vi "01 Dryer Start Stop SM.vi"() -> ()   [LabVIEW 2012]
uses:
  Dryer Com Port Info.ctl
  Dryer Status Ctrl.ctl
  StartStop Data.ctl
  GEA2 Driver/GEA2 Dryer Interface Ctrl.ctl
  <vilib>/DAQmx/read.llb/DAQmx Read (Analog 2D DBL NChan NSamp).vi
  <vilib>/DAQmx/write.llb/DAQmx Write (Digital U32 1Chan 1Samp).vi
  <vilib>/DAQmx/create/channels.llb/DAQmx Create Channel (AI-Voltage-Basic).vi
  <vilib>/DAQmx/configure/timing.llb/DAQmx Timing (Sample Clock).vi
  <vilib>/DAQmx/miscellaneous.llb/DAQmx Fill In Error Info.vi
  Globals SS.vi
  <vilib>/DAQmx/create/channels.llb/DAQmx Create Channel (DO-Digital Output).vi
  <vilib>/Utility/file.llb/Read From Spreadsheet File (DBL).vi
  <vilib>/Utility/file.llb/Write To Spreadsheet File (string).vi
  <vilib>/Utility/file.llb/Write To Spreadsheet File (DBL).vi
panel:
  in  "Tab Control":T1(tab)=enum."Raw Data"
  in  "D Data 2":dbl[](array[numeric])=[0.06788055309111314, 0.06788055309111314, 0.06788055309111314, 0.06788055309111314, 0.06788055309111314, 0.06788055309111314, 0.06788055309111314, 0.06788055309111314, 0.06788055309111314, 0.06788055309111314, 0.06788055309111314, 0.06788055309111314, 0.06788055309111314, 0.06788055309111314, 0.06788055309111314]
  in  "A Data 2":dbl[](array[numeric])
  in  "A Data":dbl[](array[numeric])
  in  "B Data":dbl[](array[numeric])
  in  "B Data 2":dbl[](array[numeric])
  in  "C Data 2":dbl[](array[numeric])
  in  "C Data":dbl[](array[numeric])
  in  "D Data":dbl[](array[numeric])=[5.851428694297497, 3.661927497414327, 3.661927497414327, 3.661927497414327, 3.661927497414327, 3.661927497414327, 3.661927497414327, 3.661927497414327, 3.661927497414327, 0.6577281807606751, 0.09762322341846881, 0.09762322341846881, 0.09762322341846881, 0.09762322341846881, 0.09762322341846881]
  in  "A save":dbl[](array[numeric])
  in  "C save":dbl[](array[numeric])
  in  "B save":dbl[](array[numeric])
  in  "D save":dbl[](array[numeric])=[5.851428694297497, 3.661927497414327, 3.661927497414327, 3.661927497414327, 3.661927497414327, 3.661927497414327, 3.661927497414327, 3.661927497414327, 3.661927497414327, 0.6577281807606751, 0.09762322341846881, 0.09762322341846881, 0.09762322341846881, 0.09762322341846881, 0.09762322341846881]
  out "Waveform Chart":dbl(graph)=0.09762322341846881
  in  "Channel":i32=6
  out "Currents":dbl[](array[numeric])=[0.0012165306634386985, -0.006587335189708488, 0.00045533310115012174, 0.009590983127054642, 0.09094609304713201, 0.048033305281516, 0.09762322341846881, 0.06788055309111314] format="%0.2f"
  in  "AI Task":refnum<k21>
  in  "Maximum Value":dbl=10.0 format="%0.2f"
  in  "Minimum Value":dbl=-10.0 format="%0.2f"
  in  "Rate":dbl=2.0 caption="Sample Rate (Hz)" format="%0.2f"
  in  "Samples per Channel":i32=1
  out "data":dbl[][](array[numeric])=[[0.0002433061326877397], [-0.0013174670379416976], [9.106662023002435e-05], [0.0019181966254109284], [0.018189218609426402], [0.0096066610563032], [0.019524644683693762], [0.013576110618222628]] format="%0.2f"
  in  "AI Channel":string="Dev2/ai0:7"
  out "Current State":string="Exit"
  out "Saving":errorcluster
  out "Stop":bool=TRUE
  out "Read Serial Count":dbl=792.0
  out "Log Coms Array":string[](array[string])=["COM2,3/1/2012,10:47:12 AM,No Com", "COM3,3/1/2012,10:47:12 AM,No Com", "COM4,3/1/2012,10:47:12 AM,No Com", "COM5,3/1/2012,10:47:12 AM,"]
  out "Status Array Out":T2[](array[typedef])=[{"Color"=0, "Last Read Status"=enum."Err", "Command:Data"="No Com", "Com Port"=2, "Time(S)"=158.546875, "Err Count"=233}, {"Color"=0, "Last Read Status"=enum."Err", "Command:Data"="No Com", "Com Port"=3, "Time(S)"=158.546875, "Err Count"=233}, {"Color"=0, "Last Read Status"=enum."Err", "Command:Data"="No Com", "Com Port"=4, "Time(S)"=158.5625, "Err Count"=233}, {"Color"=6618880, "Last Read Status"=enum."Cycle Running", "Command:Data"="", "Com Port"=5, "Time(S)"=158.5625, "Err Count"=1}]
  out "Rising Edge Out":bool[](array[boolean])
  in  "Power":bool[](array[boolean])=[FALSE, FALSE, FALSE, FALSE]
  in  "Power Port":tag="Dev2/port0" caption="Port"
  out "Restart Err Count":dbl=1.0
  in  "Cycle Save Multiple":i16=25
  out "Com Er Mess":string="Send Restart"
  out "Label Com Array":string[][](array[string])=[["Dryer A", "2"], ["Dryer B", "3"], ["Dryer C", "4"], ["Dryer D", "5"]]
  out "Current Filename":path=path "C:/Data/20120301_10_CONWAY-E5500.appl.ge.com_Dryer A_SS_Data.csv"
  in  "Timeout":i32=500
  in  "Config File":path=path "C:/data/SS_Config.ini"
  in  "Save File Path":path=path "C:/Data/Start Stop"
  out "robo?":bool
  out "Computer Name":string="CONWAY-E5500.appl.ge.com"
  in  "Cycle Count Path":path=path "c:/Data/CycleCount.csv"
  in  "Backup Hour":string="4"
  in  "Up Lim":dbl[](array[numeric])=[50.0, 50.0, 50.0, 50.0, 50.0, 4.4, 4.4, 50.0, 50.0, 50.0, 50.0, 1.0, 1.0, 1.0, 50.0, 50.0, 50.0, 50.0, 50.0, 50.0, 27.0, 27.0, 27.0, 27.0, 27.0, 27.0, 27.0, 27.0, 1.0, 1.0, 1.0, 1.0]
  in  "Low Lim 2":dbl[](array[numeric])=[-1.0, -1.0, -1.0, -1.0, -1.0, 3.5, 3.5, -1.0, -1.0, -1.0, -1.0, -1.0, -1.0, -1.0, -1.0, -1.0, -1.0, -1.0, -1.0, -1.0, -1.0, -1.0, -1.0, 22.0, -1.0, -1.0, -1.0, -1.0, -1.0, -1.0, -1.0, -1.0]
  in  "Low Lim":dbl[](array[numeric])=[-1.0, -1.0, -1.0, -1.0, -1.0, 3.5, 3.5, -1.0, -1.0, -1.0, -1.0, -1.0, -1.0, -1.0, -1.0, -1.0, -1.0, -1.0, -1.0, -1.0, -1.0, -1.0, 22.0, -1.0, -1.0, -1.0, -1.0, -1.0, -1.0, -1.0, -1.0, -1.0]
  in  "Off On Threshold":dbl=1.0
  in  "Filename Currents":path=path "c:/Data/Currents.csv"
  out "Max Len":i32
  out "A Array":string[][](array[string])
  out "B Array":string[][](array[string])
  out "D Array":string[][](array[string])=[["Dryer D,COM5,3/1/2012,10:46:45 AM,0x72:0x03\r0x72:0x03\r\nInner Coil OFF\r\nOuter Coil Relay OFF\r\nMachine EOCStep ID: 0006\r\n\r\nDrum Relay OFFCF Switch:0000"], [""], [""], [""], [""], [""], [""], ["Dryer D,COM5,3/1/2012,10:46:49 AM,0x72:0x01\r0x72:0x01\r\nMachine RunElec HS - Inlet Set Point 1 : 0330\r\nElec HS - Outlet Set Point 1 : 0135\r\nElec HS - Inlet Set Point 2: 0000\r\nElec HS - Outlet Set Point 2 : 0000\r\nElec HS - Inlet Set Point 3: 0350\r\nElec HS - Outlet Set Point 3 : 0140\r\n\r\nCurrent primitive: TimeDryStep ID: 0002\r\nBase Cycle Index: 0006\r\nEst Cycle Time In Min: 0001\r\n\r\nStart Tumble\r\nTumble"], ["Dryer D,COM5,3/1/2012,10:46:49 AM,StepID:0000\r\nCWDuration:0005\r\nStartDrum\r\nReverse Tumble set for CW\r\nDrum Relay ON\r\nCF Switch:0001\r\nDrum Started Ack\r\n1022  7113  0093  0138\r\nHtr Inh = 0004"], [""], ["Dryer D,COM5,3/1/2012,10:46:50 AM,1023  7113  0093  0138"], [""], ["Dryer D,COM5,3/1/2012,10:46:51 AM,1023  7113  0093  0138"], [""], ["Dryer D,COM5,3/1/2012,10:46:52 AM,1022  7113  0093  0139\r\n\r\nHeaterOffDuration:0000\r\nTumbleStepID:0001\r\nDrum Relay OFFReverse Tumble set for CCW"], ["Dryer D,COM5,3/1/2012,10:46:53 AM,CF Switch:0000"], ["Dryer D,COM5,3/1/2012,10:46:54 AM,1020  7113  0092  0139\r\n\r\nDrum Stop Ack\r\nCW Pause Duraiton:3000\r\nTumble Pause"], ["Dryer D,COM5,3/1/2012,10:46:54 AM,1022  7113  0092  0139"], [""], ["Dryer D,COM5,3/1/2012,10:46:55 AM,1022  7113  0093  0138"], [""], ["Dryer D,COM5,3/1/2012,10:46:56 AM,1023  7113  0093  0139\r\n\r\nTumbleStepID:0002\r\nCCWDurat"], ["Dryer D,COM5,3/1/2012,10:46:57 AM,ion:0005\r\nStartDrum\r\nDrum Relay ON\r\nCF Switch:0001"], ["Dryer D,COM5,3/1/2012,10:46:57 AM,1020  7113  0093  0139\r\nDrum Started Ack"], [""], ["Dryer D,COM5,3/1/2012,10:46:59 AM,1019  7113  0093  0139\r\nHtr Inh = 0000\r\nOuter Coil ON\r\nInner Coil ON"], ["Dryer D,COM5,3/1/2012,10:46:59 AM,1023  7113  0093  0139\r\nER1-ON \r\nER2-ON"], [""], ["Dryer D,COM5,3/1/2012,10:47:00 AM,1023  7113  0093  0139\r\n\r0x72:0x03\r0x72:0x03\r\nInner Coil OFF\r\nOuter Coil"], ["Dryer D,COM5,3/1/2012,10:47:01 AM,Relay OFF\r\nMachine EOCStep ID: 0006\r\n\r\nDrum Relay OFFCF Switch:0000"], [""], [""], [""], [""], [""], [""], ["Dryer D,COM5,3/1/2012,10:47:05 AM,0x72:0x01\r0x72:0x01\r\nMachine RunElec HS - Inlet  Outlet Set Point 1 : 0135\r\nElec HS - Inlet Set Point 2: 0000\r\nElec HS - Outlet Set Point 2 : 0000\r\nElec HS - Inlet Set Point 3: 0350\r\nElec HS - Outlet Set Point 3 : 0140\r\n\r\nCurrent primitive: TimeDryStep ID: 0002\r\nBase Cycle Index: 0006\r\nEst Cycle Time In Min: 0001\r\n\r\nStart Tumble\r\nTumbleStepID:0000\r\nCWDuration:0005"], ["Dryer D,COM5,3/1/2012,10:47:05 AM,t for CW\r\nDrum Relay ON\r\nCF Switch:0001\r\nDrum Started Ack\r\n1023  7113  0093  0139\r\nHtr Inh = 0004"], [""], ["Dryer D,COM5,3/1/2012,10:47:06 AM,1019  7113  0093  0139"], ["Dryer D,COM5,3/1/2012,10:47:07 AM,0x72:0x01\r0x72:0x01"], ["Dryer D,COM5,3/1/2012,10:47:08 AM,1021  7113  0094  0138"], [""], ["Dryer D,COM5,3/1/2012,10:47:09 AM,1021  7113  0093  0139"], ["Dryer D,COM5,3/1/2012,10:47:09 AM,HeaterOffDuration:0000\r\nTum"], ["Dryer D,COM5,3/1/2012,10:47:10 AM,bleStepID:0001\r\nDrum Relay OFFReverse Tumble set for CCW\r\n1020  7113  0094  0139\r\nCF Switch:0000"], ["Dryer D,COM5,3/1/2012,10:47:10 AM,1021  7113  0094  0139\r\n\r\nDrum Stop Ack\r\nCW Pause Dur"], ["Dryer D,COM5,3/1/2012,10:47:11 AM,aiton:3000\r\nTumble Pause"], ["Dryer D,COM5,3/1/2012,10:47:12 AM,1023  7113  0094  0139"], [""]]
  out "C Array":string[][](array[string])
  out "Ready":bool=TRUE
  in  "Change Lint":bool
  out "Station D: L1 Current":waveform(dbl)[](graph)=[{"t0"=timestamp(0 s since 1904-01-01), "dt"=0.5, "Y"=[50.0, 50.0, 50.0, 50.0, 50.0, 4.4, 4.4, 50.0, 50.0, 50.0, 50.0, 1.0, 1.0, 1.0, 50.0, 50.0, 50.0, 50.0, 50.0, 50.0, 27.0, 27.0, 27.0, 27.0, 27.0, 27.0, 27.0, 27.0, 1.0, 1.0, 1.0, 1.0]}, {"t0"=timestamp(0 s since 1904-01-01), "dt"=0.5, "Y"=[-1.0, -1.0, -1.0, -1.0, -1.0, 3.5, 3.5, -1.0, -1.0, -1.0, -1.0, -1.0, -1.0, -1.0, -1.0, -1.0, -1.0, -1.0, -1.0, -1.0, -1.0, -1.0, 22.0, -1.0, -1.0, -1.0, -1.0, -1.0, -1.0, -1.0, -1.0, -1.0]}, {"t0"=timestamp(0 s since 1904-01-01), "dt"=0.5, "Y"=[5.851428694297497, 3.661927497414327, 3.661927497414327, 3.661927497414327, 3.661927497414327, 3.661927497414327, 3.661927497414327, 3.661927497414327, 3.661927497414327, 0.6577281807606751, 0.09762322341846881, 0.09762322341846881, 0.09762322341846881, 0.09762322341846881, 0.09762322341846881]}, {"t0"=timestamp(0 s since 1904-01-01), "dt"=0.5, "Y"=[0.06788055309111314, 0.06788055309111314, 0.06788055309111314, 0.06788055309111314, 0.06788055309111314, 0.06788055309111314, 0.06788055309111314, 0.06788055309111314, 0.06788055309111314, 0.06788055309111314, 0.06788055309111314, 0.06788055309111314, 0.06788055309111314, 0.06788055309111314, 0.06788055309111314]}, {"t0"=timestamp(0 s since 1904-01-01), "dt"=0.5, "Y"=[-1.0, -1.0, -1.0, -1.0, -1.0, 3.5, 3.5, -1.0, -1.0, -1.0, -1.0, -1.0, -1.0, -1.0, -1.0, -1.0, -1.0, -1.0, -1.0, -1.0, -1.0, -1.0, -1.0, 22.0, -1.0, -1.0, -1.0, -1.0, -1.0, -1.0, -1.0, -1.0]}]
  out "Station B: L1 Current":waveform(dbl)[](graph)=[{"t0"=timestamp(0 s since 1904-01-01), "dt"=0.5, "Y"=[50.0, 50.0, 50.0, 50.0, 50.0, 4.4, 4.4, 50.0, 50.0, 50.0, 50.0, 1.0, 1.0, 1.0, 50.0, 50.0, 50.0, 50.0, 50.0, 50.0, 27.0, 27.0, 27.0, 27.0, 27.0, 27.0, 27.0, 27.0, 1.0, 1.0, 1.0, 1.0]}, {"t0"=timestamp(0 s since 1904-01-01), "dt"=0.5, "Y"=[-1.0, -1.0, -1.0, -1.0, -1.0, 3.5, 3.5, -1.0, -1.0, -1.0, -1.0, -1.0, -1.0, -1.0, -1.0, -1.0, -1.0, -1.0, -1.0, -1.0, -1.0, -1.0, 22.0, -1.0, -1.0, -1.0, -1.0, -1.0, -1.0, -1.0, -1.0, -1.0]}, {"t0"=timestamp(0 s since 1904-01-01), "dt"=0.5, "Y"=[]}, {"t0"=timestamp(0 s since 1904-01-01), "dt"=0.5, "Y"=[]}, {"t0"=timestamp(0 s since 1904-01-01), "dt"=0.5, "Y"=[-1.0, -1.0, -1.0, -1.0, -1.0, 3.5, 3.5, -1.0, -1.0, -1.0, -1.0, -1.0, -1.0, -1.0, -1.0, -1.0, -1.0, -1.0, -1.0, -1.0, -1.0, -1.0, -1.0, 22.0, -1.0, -1.0, -1.0, -1.0, -1.0, -1.0, -1.0, -1.0]}]
  out "Station C: L1 Current":waveform(dbl)[](graph)=[{"t0"=timestamp(0 s since 1904-01-01), "dt"=0.5, "Y"=[50.0, 50.0, 50.0, 50.0, 50.0, 4.4, 4.4, 50.0, 50.0, 50.0, 50.0, 1.0, 1.0, 1.0, 50.0, 50.0, 50.0, 50.0, 50.0, 50.0, 27.0, 27.0, 27.0, 27.0, 27.0, 27.0, 27.0, 27.0, 1.0, 1.0, 1.0, 1.0]}, {"t0"=timestamp(0 s since 1904-01-01), "dt"=0.5, "Y"=[-1.0, -1.0, -1.0, -1.0, -1.0, 3.5, 3.5, -1.0, -1.0, -1.0, -1.0, -1.0, -1.0, -1.0, -1.0, -1.0, -1.0, -1.0, -1.0, -1.0, -1.0, -1.0, 22.0, -1.0, -1.0, -1.0, -1.0, -1.0, -1.0, -1.0, -1.0, -1.0]}, {"t0"=timestamp(0 s since 1904-01-01), "dt"=0.5, "Y"=[]}, {"t0"=timestamp(0 s since 1904-01-01), "dt"=0.5, "Y"=[]}, {"t0"=timestamp(0 s since 1904-01-01), "dt"=0.5, "Y"=[-1.0, -1.0, -1.0, -1.0, -1.0, 3.5, 3.5, -1.0, -1.0, -1.0, -1.0, -1.0, -1.0, -1.0, -1.0, -1.0, -1.0, -1.0, -1.0, -1.0, -1.0, -1.0, -1.0, 22.0, -1.0, -1.0, -1.0, -1.0, -1.0, -1.0, -1.0, -1.0]}]
  out "Station A: L1 Current":waveform(dbl)[](graph)=[{"t0"=timestamp(0 s since 1904-01-01), "dt"=0.5, "Y"=[50.0, 50.0, 50.0, 50.0, 50.0, 4.4, 4.4, 50.0, 50.0, 50.0, 50.0, 1.0, 1.0, 1.0, 50.0, 50.0, 50.0, 50.0, 50.0, 50.0, 27.0, 27.0, 27.0, 27.0, 27.0, 27.0, 27.0, 27.0, 1.0, 1.0, 1.0, 1.0]}, {"t0"=timestamp(0 s since 1904-01-01), "dt"=0.5, "Y"=[-1.0, -1.0, -1.0, -1.0, -1.0, 3.5, 3.5, -1.0, -1.0, -1.0, -1.0, -1.0, -1.0, -1.0, -1.0, -1.0, -1.0, -1.0, -1.0, -1.0, -1.0, -1.0, 22.0, -1.0, -1.0, -1.0, -1.0, -1.0, -1.0, -1.0, -1.0, -1.0]}, {"t0"=timestamp(0 s since 1904-01-01), "dt"=0.5, "Y"=[]}, {"t0"=timestamp(0 s since 1904-01-01), "dt"=0.5, "Y"=[]}, {"t0"=timestamp(0 s since 1904-01-01), "dt"=0.5, "Y"=[-1.0, -1.0, -1.0, -1.0, -1.0, 3.5, 3.5, -1.0, -1.0, -1.0, -1.0, -1.0, -1.0, -1.0, -1.0, -1.0, -1.0, -1.0, -1.0, -1.0, -1.0, -1.0, -1.0, 22.0, -1.0, -1.0, -1.0, -1.0, -1.0, -1.0, -1.0, -1.0]}]
  out "Read_ACK":bool=TRUE
  in  "Init":bool
  out "Reading":bool
  in  "Select Station":string(combo)="Dryer D"
  in  "Command:Data":string=" 7111  0087  0114\r\n\n--------------------\n1023  7111  0087  0114\r\n\n--------------------\n1023  7111  0087  0116\r\n\n--------------------\n\r\nHeaterOffDuration:0000\r\nTumbleStepID:0001\r\nDrum Relay OFFReverse Tumble set for CCW\r\n\n--------------------\nCF Switch:0000\r\n1023  7111  0087  0116\r\n\n--------------------\n\r\nDrum Stop Ack\r\nCW Pause Duraiton:3000\r\nTumble Pause\n--------------------\n1023  7111  0087  0116\r\n\n--------------------\n1023  7111  0087  0118\r\n\n--------------------\n1022  7111  0087  0118\r\n\n--------------------\n\r\nTumbleStepID:0002\r\nCCWDuration:0005\r\nStartDrum\r\nDrum Relay ON\r\nCF Switch:0001\r\n1023  7111  0087  0120\r\n\n--------------------\nDrum Started Ack\r\n\n--------------------\n1023  7111  0087  0119\r\nHtr Inh = 0000\r\nOuter Coil ON\r\nInner Coil ON\r\n\n--------------------\n1023  7111  0088  0120\r\nER1-ON \r\nER2-ON \r\n\n--------------------\n1023  7111  0088  0120\r\n\r0x72:0x03\r0x72:0x03\r\nInner Coil OFF\r\nOuter Coil \n--------------------\nRelay OFF\r\nMachine EOCStep ID: 0006\r\n\r\nDrum Relay OFFCF Switch:0000\r\n\n--------------------\n0x72:0x01\r0x72:0x01\r\nMachine RunElec HS - Inlet Set Point 1 : 0330\r\nElec HS - Outlet Set Point 1 : 0135\r\nElec HS - Inlet Set Point 2: 0000\r\nElec HS - Outlet Set Point 2 : 0000\r\nElec HS - Inlet Set Point 3: 0350\r\nElec HS - Outlet Set Point 3 : 0140\r\n\r\nCurrent primitive: TimeDryStep ID: 0002\r\nBase Cycle Index: 0006\r\nEst Cycle Time In Min: 0001\r\n\r\nStart Tumble\r\nTumble\n--------------------\nStepID:0000\r\nCWDuration:0005\r\nStartDrum\r\nReverse Tumble set for CW\r\nDrum Relay ON\r\nCF Switch:0001\r\nDrum Started Ack\r\n1022  7111  0088  0123\r\nHtr Inh = 0004\n--------------------\n1023  7111  0088  0123\r\n\n--------------------\n1023  7111  0088  0124\r\n\n--------------------\n1023  7111  0088  0124\r\n\n--------------------\n\r\nHeaterOffDuration:0000\r\nTum\n--------------------\nbleStepID:0001\r\nDrum Relay OFFReverse Tumble set for CCW\r\n1023  7111  0088  0125\r\nCF Switch:0000\r\n\n--------------------\n1023  7111  0088  0124\r\n\r\nDrum Stop Ack\r\nCW Pause Dur\n--------------------\naiton:3000\r\nTumble Pause\n--------------------\n1021  7111  0088  0125\r\n\n--------------------\n1023  7111  0088  0126\r\n\n--------------------\n1023  7111  0089  0126\r\n\r\nTumbleStepID:0002\r\nCCWDuration:0005\r\nStartDrum\r\nDrum Relay ON\r\n\n--------------------\nCF Switch:0001\r\n1023  7111  0088  0126\r\n\n--------------------\nDrum Started Ack\r\n\n--------------------\n1023  7111  0089  0126\r\nHtr Inh = 0000\r\nOuter Coil ON\r\nInner Coil ON\r\n\n--------------------\n1023  7111  0089  0127\r\nER1-ON \r\nER2-ON \r\n\n--------------------\n0x72:0x03\r0x72:0x03\r\nInner Coil OFF\r\nOuter Coil Relay OFF\r\nMachine EOCStep ID: 0006\r\n\r\nDrum Relay OFFCF Switch:0000\r\n\n--------------------\n0x72:0x01\r0x72:0x01\r\nMachine RunElec HS - Inlet Set Point 1 : 0330\r\nElec HS - Outlet Set Point 1 : 0135\r\nElec HS - Inlet Set Point 2: 0000\r\nElec HS - Outlet Set Point 2 : 0000\r\nElec HS - Inlet Set Point 3: 0350\r\nElec HS - Outlet Set Point 3 : 0140\r\n\r\nCurrent primitive: TimeDryStep ID: 0002\r\nBase Cycle Index: 0006\r\nEst Cycle Time In Min: 0001\r\n\r\nStart Tumble\r\nTumble\n--------------------\nStepID:0000\r\nCWDuration:0005\r\nStartDrum\r\nReverse Tumble set for CW\r\nDrum Relay ON\r\nCF Switch:0001\r\nDrum Started Ack\r\n1023  7111  0089  0127\r\nHtr Inh = 0004\n--------------------\n1023  7111  0089  0128\r\n\n--------------------\n1023  7111  0089  0127\r\n\n--------------------\n1023  7111  0089  0127\r\n\n--------------------\n\r\nHeaterOffDuration:0000\r\nTumbleStepID:0001\r\nDrum Relay OFFReverse Tumble set for CCW\r\n\n--------------------\nCF Switch:0000\r\n1023  7111  0089  0128\r\n\n--------------------\n\r\nDrum Stop Ack\r\nCW Pause Duraiton:3000\r\nTumble Pause1023 \n--------------------\n 7111  0090  0127\r\n\n--------------------\n1023  7111  0090  0128\r\n\n--------------------\n0x72:0x01\r0x72:0x01\n--------------------\n1023  7111  0090  0128\r\n\n--------------------\n\r\nTumbleStepID:0002\r\nCCWDuration:0005\r\nStartDrum\r\nDrum Relay ON\r\n1023  7111  0090  0128\r\n\n--------------------\nCF Switch:0001\r\n\n--------------------\nDrum Started Ack\r\n1023  7111  0090  0128\r\nHtr Inh = 0000\r\nOuter Coil ON\r\nInner Coil ON\r\n\n--------------------\n1023  7111  0090  0129\r\nER1-ON \r\nER2-ON \r\n\n--------------------\n1023  7111  0090  0128\r\n\n--------------------\n0x72:0x03\r0x72:0x03\r\nInner Coil OFF\r\nOuter Coil Relay OFF\r\nMachine EOCStep ID: 0006\r\n\r\nDrum Relay OFFCF Switch:0000\r\n\n--------------------\n0x72:0x01\r0x72:0x01\r\nMachine RunElec HS - Inlet Set Point 1 : 0330\r\nElec HS - Outlet Set Point 1 : 0135\r\nElec HS - Inlet Set Point 2: 0000\r\nElec HS - Outlet Set Point 2 : 0000\r\nElec HS - Inlet Set Point 3: 0350\r\nElec HS - Outlet Set Point 3 : 0140\r\n\r\nCurrent primitive: TimeDryStep ID: 0002\r\nBase Cycle Index: 0006\r\nEst Cycle Time In Min: 0001\r\n\r\nStart Tumble\r\nTumbleStepID:0000\r\nCWDuration:0005\r\n--------------------\n\nStartDrum\r\nReverse Tumble set for CW\r\nDrum Relay ON\r\nCF Switch:0001\r\nDrum Started Ack\r\n1023  7111  0090  0129\r\nHtr Inh = 0004\n--------------------\n1023  7111  0090  0131\r\n\n--------------------\n1023  7111  0090  0130\r\n\n--------------------\n1023  7111  0090  0131\r\n\n--------------------\n\r\nHeaterOffDuration:0000\r\nTumbleStepID:0001\r\nDrum Relay OFFReverse Tumble set for CCW\r\nCF Switch:0000\r\n1023  7111  0\n--------------------\n091  0131\r\n\n--------------------\n\r\nDrum Stop Ack\r\nCW Pause Duraiton:3000\r\nTumble Pause1023  7111  0090  0131\r\n\n--------------------\n1023  7111  0091  0132\r\n\n--------------------\n1023  7111  0091  0132\r\n\n--------------------\n\r\nTumbleStepID:0002\r\nCCWDurat\n--------------------\nion:0005\r\nStartDrum\r\nDrum Relay ON\r\n1023  7111  0091  0133\r\nCF Switch:0001\r\n\n--------------------\nDrum Started Ack\r\n1022  7111  0091  0133\r\nHtr I\n--------------------\nnh = 0000\r\nOuter Coil ON\r\nInner Coil ON\r\n\n--------------------\n1023  7111  0091  0134\r\nER1-ON \r\nER2-ON \r\n\n--------------------\n1022  7111  0091  0134\r\n\n--------------------\n0x72:0x03\r0x72:0x03\r\nInner Coil OFF\r\nOuter Coil Relay OFF\r\nMachine EOCStep ID\n--------------------\n: 0006\r\n\r\nDrum Relay OFFCF Switch:0000\r\n\n--------------------\n0x72:0x01\r0x72:0x01\r\nMachine RunElec HS - Inlet  Outlet Set Point 1 : 0135\r\nElec HS - Inlet Set Point 2: 0000\r\nElec HS - Outlet Set Point 2 : 0000\r\nElec HS - Inlet Set Point 3: 0350\r\nElec HS - Outlet Set Point 3 : 0140\r\n\r\nCurrent primitive: TimeDryStep ID: 0002\r\nBase Cycle Index: 0006\r\nEst Cycle Time In Min: 0001\r\n\r\nStart Tumble\r\nTumbleStepID:0000\r\nCWDuration:0005\r\n--------------------\n\nStartDrum\r\nReverse Tumble set for CW\r\nDrum Relay ON\r\nCF Switch:0001\r\nDrum Started Ack\r\n1023  7111  0092  0134\r\nHtr Inh = 0004\n--------------------\n1022  7111  0091  0135\r\n\n--------------------\n1022  7111  0091  0135\r\n\n--------------------\n1023  7111  0092  0135\r\n\r\nHeaterOffDuration:0000\r\nTum\n--------------------\nbleStepID:0001\r\nDrum Relay OFFReverse Tumble set for CCW\r\nCF Switch:0000\r\n1020  7111  0092  0136\r\n\n--------------------\n\r\nDrum Stop Ack\r\nCW Pause Duraiton:3000\r\nTumble Pause1021  7111  0092  0136\r\n\n--------------------\n1019  7111  0092  0136\r\n\n--------------------\n1019  7111  0091  0136\r\n\n--------------------\n\r\nTumbleStepID:0002\r\nCCWDuration:0005\r\nStartDrum\r\nDrum Relay ON\r\n\n--------------------\nCF Switch:0001\r\n1022  7111  0092  0136\r\n\n--------------------\nDrum Started Ack\r\n1023  7111  0091  0137\r\nHtr I\n--------------------\nnh = 0000\r\nOuter Coil ON\r\nInner Coil ON\r\n\n--------------------\n1023  7111  0092  0138\r\nER1-ON \r\nER2-ON \r\n\n--------------------\n1023  7111  0092  0137\r\n\n--------------------\n0x72:0x03\r0x72:0x03\r\nInner Coil OFF\r\nOuter Coil Relay OFF\r\nMachine EOCStep ID: 0006\r\n\r\nDrum Relay OFFCF Switch:0000\r\n\n--------------------\n0x72:0x01\r0x72:0x01\r\nMachine RunElec HS - Inlet Set Point 1 : 0330\r\nElec HS - Outlet Set Point 1 : 0135\r\nElec HS - Inlet Set Point 2: 0000\r\nElec HS - Outlet Set Point 2 : 0000\r\nElec HS - Inlet Set Point 3: 0350\r\nElec HS - Outlet Set Point 3 : 0140\r\n\r\nCurrent primitive: TimeDryStep ID: 0002\r\nBase Cycle Index: 0006\r\nEst Cycle Time In Min: 0001\r\n\r\nStart Tumble\r\nTumble\n--------------------\nStepID:0000\r\nCWDuration:0005\r\nStartDrum\r\nReverse Tumble set for CW\r\nDrum Relay ON\r\nCF Switch:0001\r\nDrum Started Ack\r\n1022  7113  0093  0138\r\nHtr Inh = 0004\n--------------------\n1023  7113  0093  0138\r\n\n--------------------\n1023  7113  0093  0138\r\n\n--------------------\n1022  7113  0093  0139\r\n\r\nHeaterOffDuration:0000\r\nTumbleStepID:0001\r\nDrum Relay OFFReverse Tumble set for CCW\r\n\n--------------------\nCF Switch:0000\r\n\n--------------------\n1020  7113  0092  0139\r\n\r\nDrum Stop Ack\r\nCW Pause Duraiton:3000\r\nTumble Pause\n--------------------\n1022  7113  0092  0139\r\n\n--------------------\n1022  7113  0093  0138\r\n\n--------------------\n1023  7113  0093  0139\r\n\r\nTumbleStepID:0002\r\nCCWDurat\n--------------------\nion:0005\r\nStartDrum\r\nDrum Relay ON\r\nCF Switch:0001\r\n\n--------------------\n1020  7113  0093  0139\r\nDrum Started Ack\r\n\n--------------------\n1019  7113  0093  0139\r\nHtr Inh = 0000\r\nOuter Coil ON\r\nInner Coil ON\r\n\n--------------------\n1023  7113  0093  0139\r\nER1-ON \r\nER2-ON \r\n\n--------------------\n1023  7113  0093  0139\r\n\r0x72:0x03\r0x72:0x03\r\nInner Coil OFF\r\nOuter Coil \n--------------------\nRelay OFF\r\nMachine EOCStep ID: 0006\r\n\r\nDrum Relay OFFCF Switch:0000\r\n\n--------------------\n0x72:0x01\r0x72:0x01\r\nMachine RunElec HS - Inlet  Outlet Set Point 1 : 0135\r\nElec HS - Inlet Set Point 2: 0000\r\nElec HS - Outlet Set Point 2 : 0000\r\nElec HS - Inlet Set Point 3: 0350\r\nElec HS - Outlet Set Point 3 : 0140\r\n\r\nCurrent primitive: TimeDryStep ID: 0002\r\nBase Cycle Index: 0006\r\nEst Cycle Time In Min: 0001\r\n\r\nStart Tumble\r\nTumbleStepID:0000\r\nCWDuration:0005\r\n--------------------\nt for CW\r\nDrum Relay ON\r\nCF Switch:0001\r\nDrum Started Ack\r\n1023  7113  0093  0139\r\nHtr Inh = 0004\n--------------------\n1019  7113  0093  0139\r\n\n--------------------\n0x72:0x01\r0x72:0x01\n--------------------\n1021  7113  0094  0138\r\n\n--------------------\n1021  7113  0093  0139\r\n\n--------------------\n\r\nHeaterOffDuration:0000\r\nTum\n--------------------\nbleStepID:0001\r\nDrum Relay OFFReverse Tumble set for CCW\r\n1020  7113  0094  0139\r\nCF Switch:0000\r\n\n--------------------\n1021  7113  0094  0139\r\n\r\nDrum Stop Ack\r\nCW Pause Dur\n--------------------\naiton:3000\r\nTumble Pause\n--------------------\n1023  7113  0094  0139\r\n"
  in  "UI Array":T4[](array[typedef])=[{"Label"="Dryer A", "Color"=0, "Last Read Status"=enum."Err", "Command:Data"="No Com", "Err Count"=233, "Cycle Count"=0}, {"Label"="Dryer B", "Color"=0, "Last Read Status"=enum."Err", "Command:Data"="No Com", "Err Count"=233, "Cycle Count"=0}, {"Label"="Dryer C", "Color"=0, "Last Read Status"=enum."Err", "Command:Data"="No Com", "Err Count"=233, "Cycle Count"=0}, {"Label"="Dryer D", "Color"=6618880, "Last Read Status"=enum."Cycle Running", "Command:Data"="", "Err Count"=1, "Cycle Count"=9}]
  in  "Exit":bool
  out "A Alarm":bool
  out "B Alarm":bool
  out "C Alarm":bool
  out "D Alarm":bool
  # "Used for rising edge to detect start of cycle."
  # "If after its done, the power is above this\nlimit, the contactor will remove power from the\ndryer."
  # "Restarts when 2 consec samples are < Off Limit, and Above On limit.\nSamples must be below Up Lim, and above either of the Low Lims.  Does not restart between the samples Restart LL, and Restart UL.  If after an alarm, the \ncurrent is > Off Current Lim, then shuts off power."
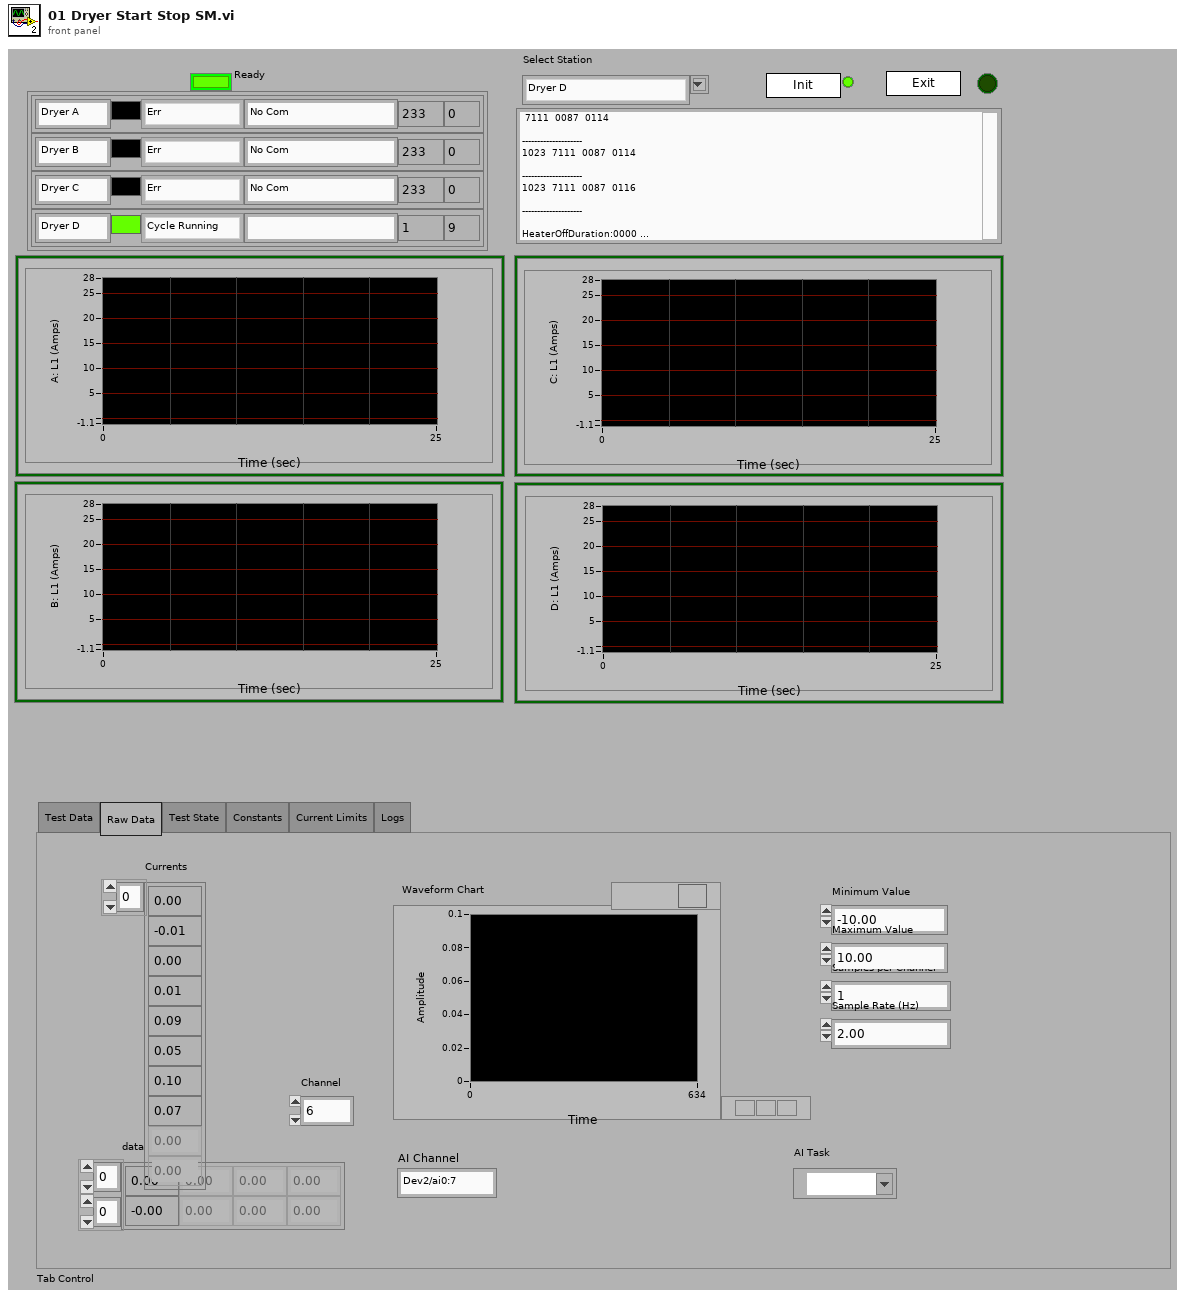
[diagram p1: front panel]
types:
  T1 = enum32{"Test Data", "Raw Data", "Test State", "Constants", "Current Limits", "Logs"}
  T2 = typedef "Dryer Com Port Info.ctl" = cluster{"Color":u32, "Last Read Status":T3, "Command:Data":string, "Com Port":u8, "Time(S)":dbl, "Err Count":u32}
  T3 = typedef "Dryer Status Ctrl.ctl" = enum16{"Cycle Not Started", "Cycle Running", "Paused", "Cycle Completed", "Eval Mode Entered", "Err"}
  T4 = typedef "StartStop Data.ctl" = cluster{"Label":string, "Color":u32, "Last Read Status":T3, "Command:Data":string, "Err Count":u32, "Cycle Count":u32}
  T5 = typedef "GEA2 Dryer Interface Ctrl.ctl" = enum16{"Init Com Port", "SendCMD", "ReadPort", "Close Port", "Simulate Diag Data", "Simulate Dryer", "Send WILT Startup CMDs", "Send Continue CMD", "Read Continuous"}
  T6 = enum32{"invalid app kind", "Development System", "Run Time System", "Student Edition", "Embedded LabVIEW", "Evaluation", "Custom"}
  T7 = enum32{"Invalid", "Standard", "Closed", "Hidden", "Minimized", "Maximized"}
  T8 = cluster{"Core":cluster{"Current VI Reference":refnum<vi>, "Close Panel on Exit?":bool}, "Data to Save":string[][], "Label Com Array":string[][], "UI Array":T4[], "Com Array":u8[], "Save File Path":path, "Last Hour":string, "Computer Name":string, "task out":refnum<k21>, "Power":bool[]}
  T9 = cluster{"Current VI Reference":refnum<vi>, "Close Panel on Exit?":bool}
  T10 = cluster{"A Alarm":bool, "B Alarm":bool, "C Alarm":bool, "D Alarm":bool}
  T11 = cluster{"Waveform":dbl, "Waveform":dbl, "Waveform":dbl, "Waveform":dbl}
  T12 = cluster{"Alatch":bool, "Blatch":bool, "Clatch":bool, "Dlatch":bool, "AI Task":refnum<k21>, "A Data":dbl[], "A Data2":dbl[], "B Data":dbl[], "B Data2":dbl[], "C Data":dbl[], "C Data2":dbl[], "D Data":dbl[], "D Data2":dbl[], "Read Data":dbl[], "Old Data":dbl[], "Rise":bool[]}
  T13 = cluster{"Rise[0]":bool, "Rise[1]":bool, "Rise[2]":bool, "Rise[3]":bool}
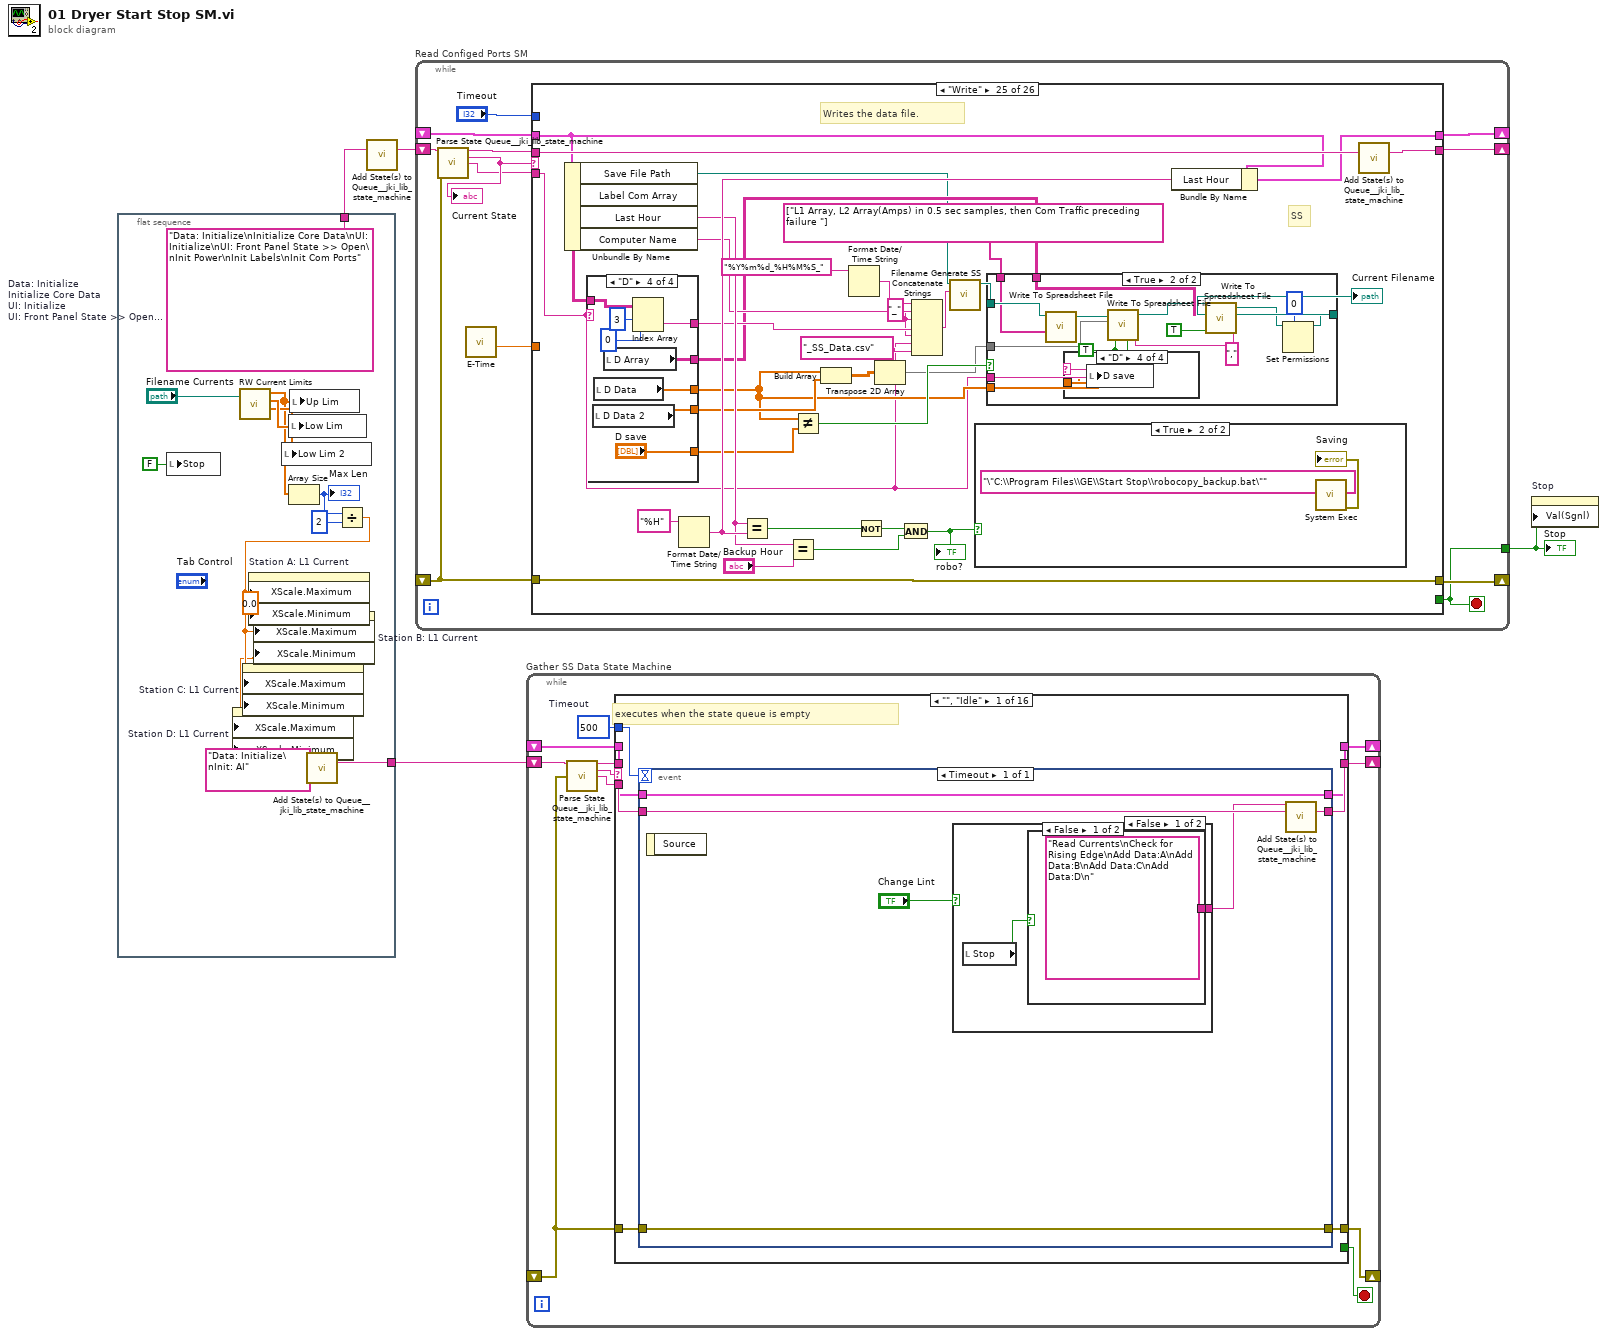
[diagram p0: block diagram]
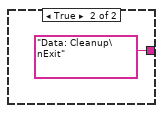
[diagram p2: hidden frame]
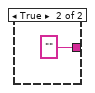
[diagram p3: hidden frame]
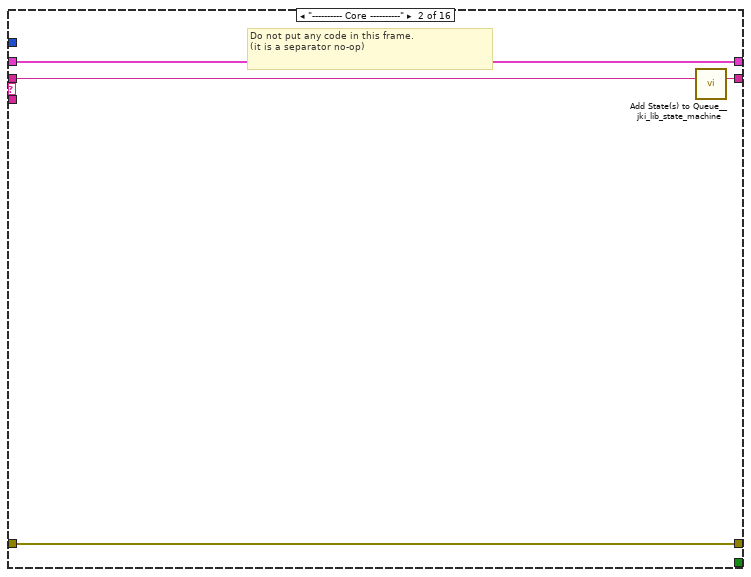
[diagram p4: hidden frame]
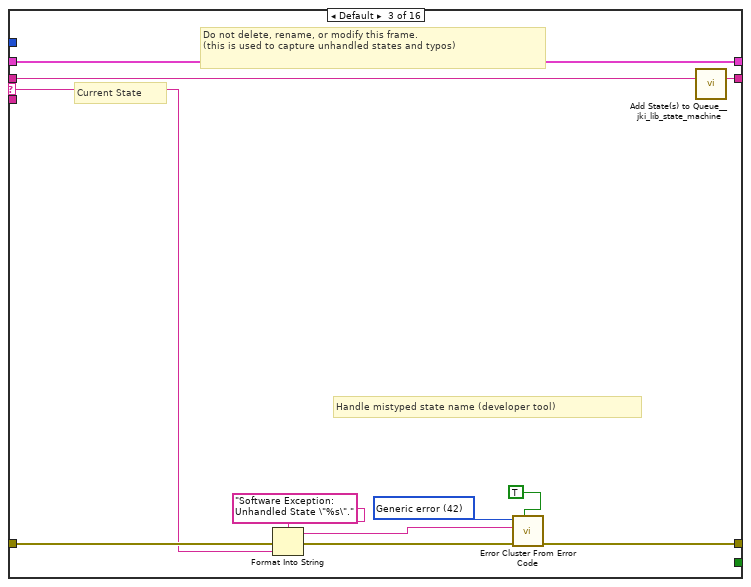
[diagram p5: hidden frame]
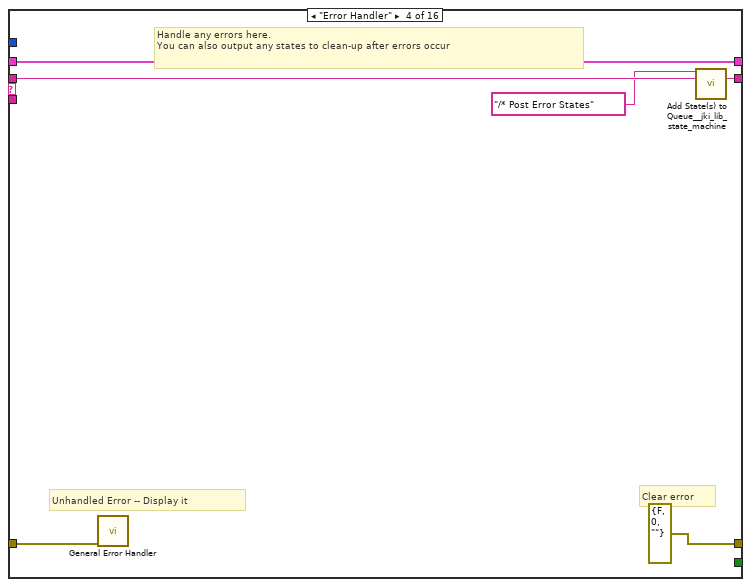
[diagram p6: hidden frame]
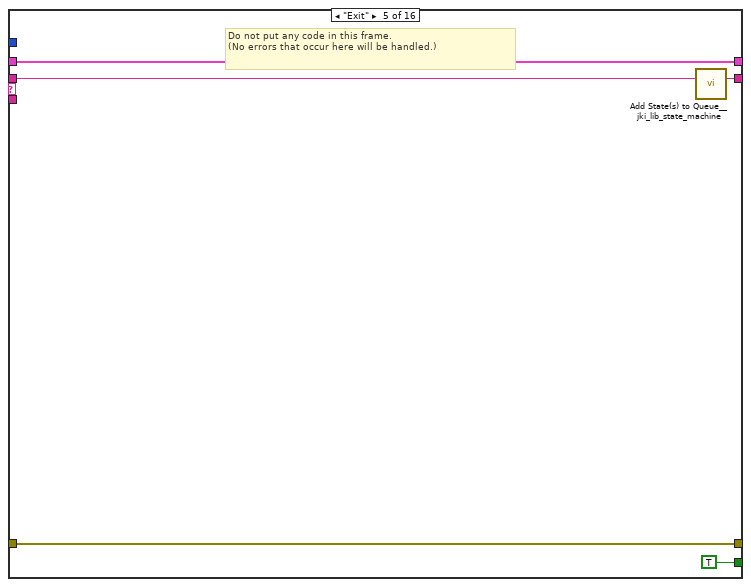
[diagram p7: hidden frame]
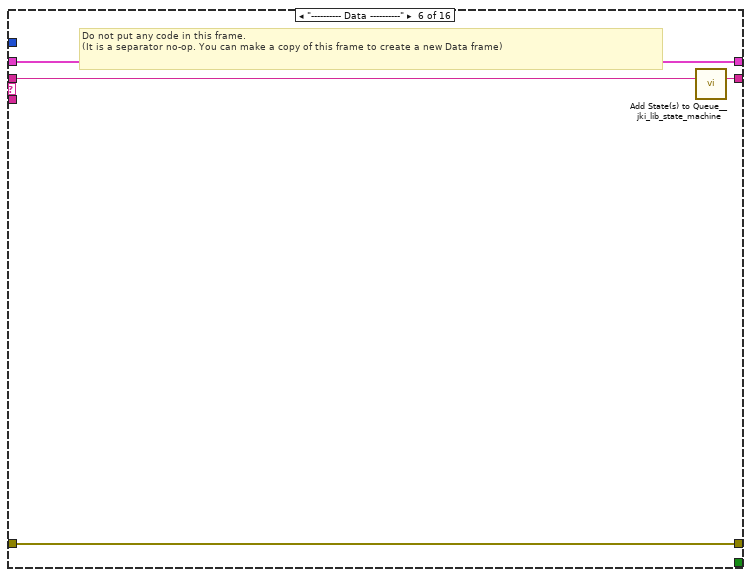
[diagram p8: hidden frame]
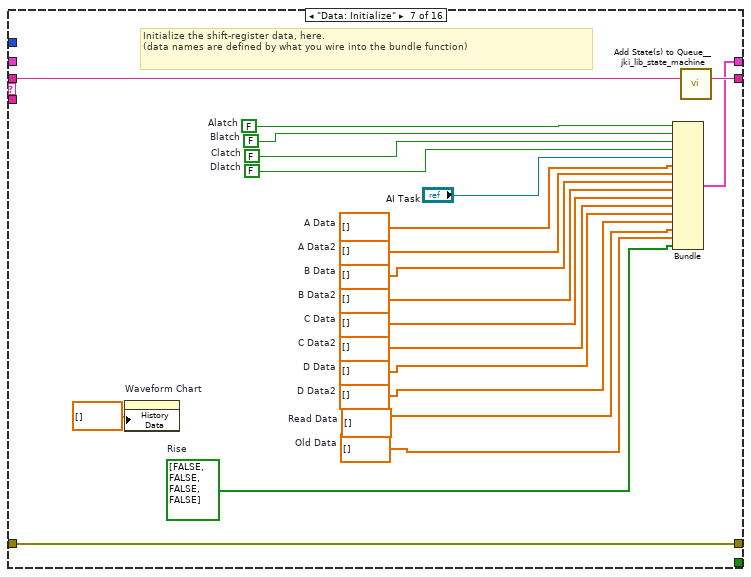
[diagram p9: hidden frame]
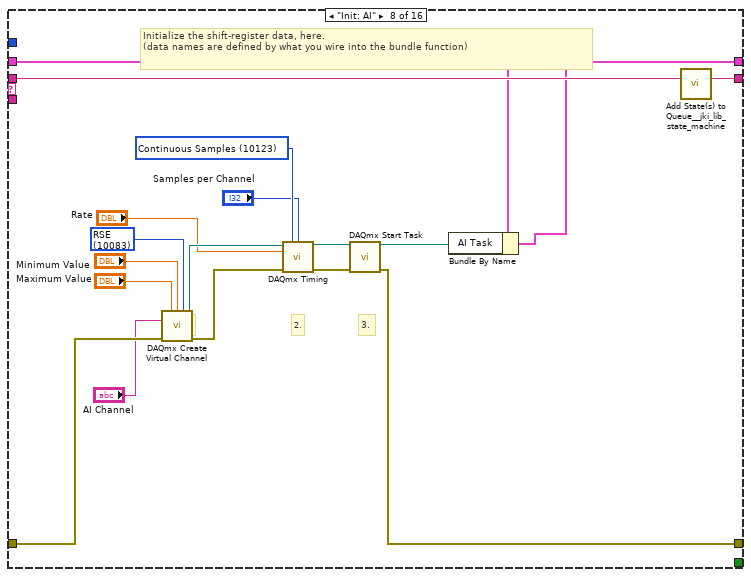
[diagram p10: hidden frame]
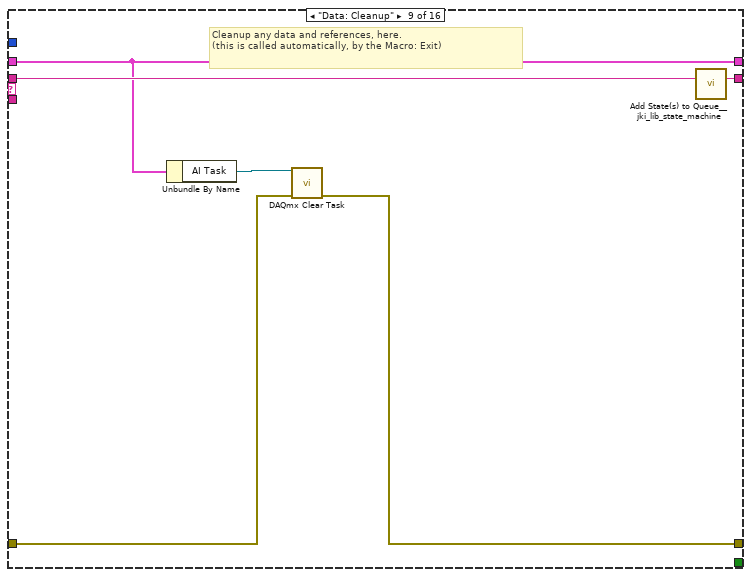
[diagram p11: hidden frame]
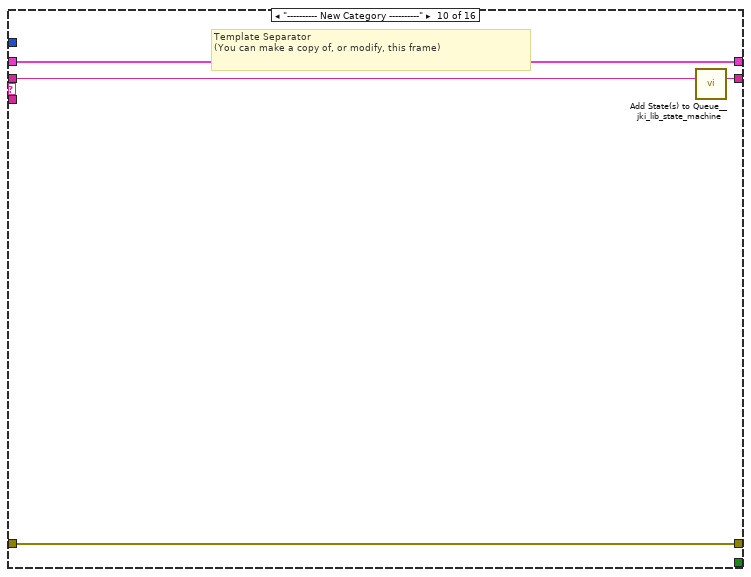
[diagram p12: hidden frame]
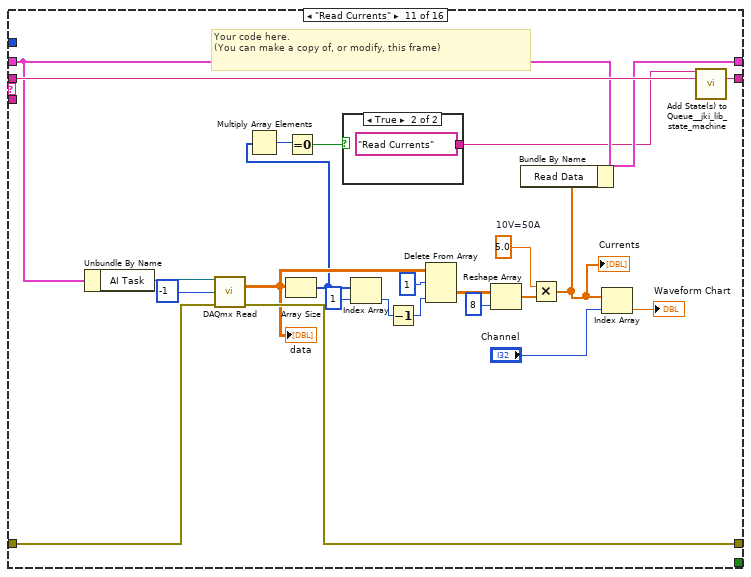
[diagram p13: hidden frame]
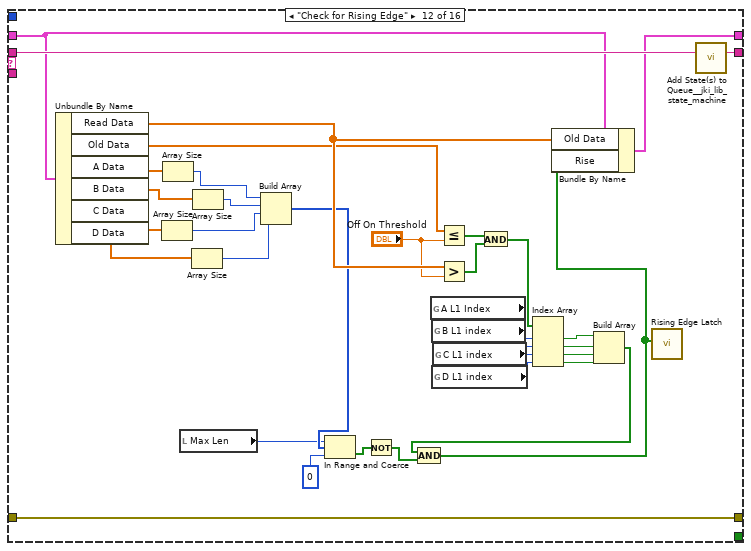
[diagram p15: hidden frame]
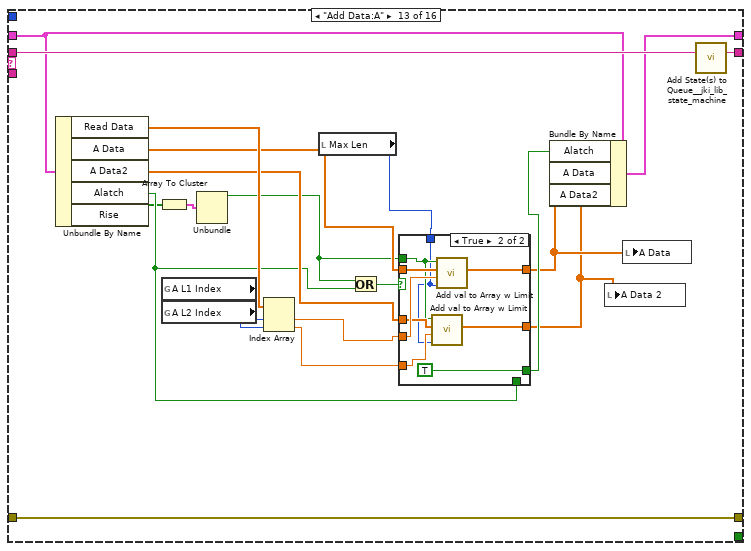
[diagram p16: hidden frame]
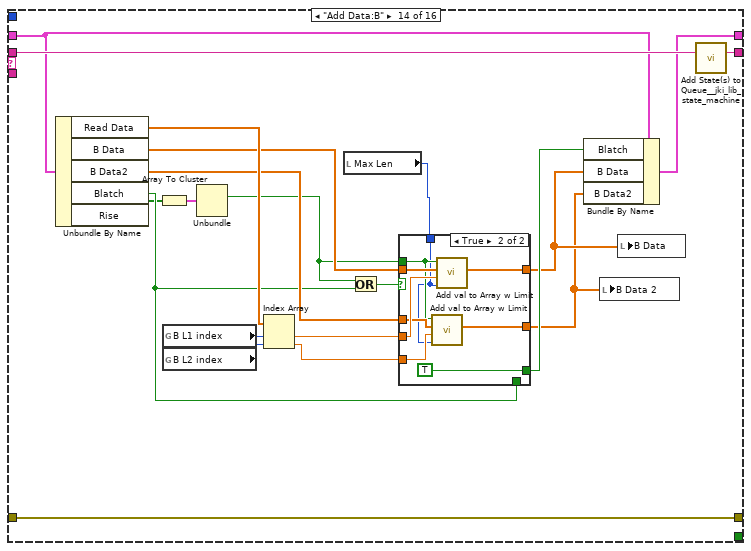
[diagram p18: hidden frame]
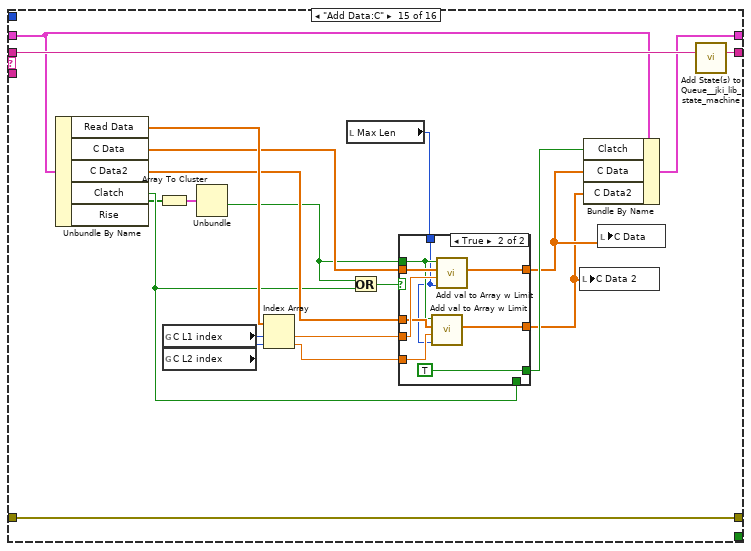
[diagram p20: hidden frame]
diagram:
  n1 = flat-sequence {
    tunnel: [w16] -> w2
    tunnel: [w15] -> w1
    frame #0 {
      w5 = 0.0 ("X Scale.Range:Minimum")
      w16 = "Data: Initialize\nInitialize Core Data\nUI: Initialize\nUI: Front Panel State >> Open\nInit Power\nInit Labels\nInit Com Ports"  # Data: Initialize Initialize Core Data UI: Initialize UI: Front Panel State >> Open Init Power Init Labels Init Com Ports
      n2 = local write "Stop"(FALSE ("Stop")) -> ()
      n3 = call "RW Current Limits.vi"("file path (dialog if empty)"="Filename Currents") -> ("Low Lim 2 Out"=w10:dbl[], "Low Lim Out"=w11:dbl[], "Up Lim Out"=w9:dbl[])  [unwired: 8 in]
      n4 = local write "Low Lim 2"(w10) -> ()
      n5 = local write "Low Lim"(w11) -> ()
      n6 = Array Size(array=w9) -> (size(s)=w8:i32)
      "Max Len" <- w8
      n7 = local write "Up Lim"(w9) -> ()
      n8 = call <vilib>:"Add State(s) to Queue__jki_lib_state_machine.vi"("State(s) in (\"\")"="Data: Initialize\nInit: AI") -> ("States Out"=w15:string)  [unwired: 14 in]
      n9 = Divide(x=w8, y=2) -> (x/y=w6:dbl)
      n10 = property on="Station D: L1 Current" class="WFChart (strict)"("XScale.Maximum"=w6, "XScale.Minimum"=w5) -> ()  [unwired: 2 in, 2 out]
      n11 = property on="Station C: L1 Current" class="WFChart (strict)"("XScale.Maximum"=w6, "XScale.Minimum"=w5) -> ()  [unwired: 2 in, 2 out]
      n12 = property on="Station A: L1 Current" class="WFChart (strict)"("XScale.Maximum"=w6, "XScale.Minimum"=w5) -> ()  [unwired: 2 in, 2 out]
      n13 = property on="Station B: L1 Current" class="WFChart (strict)"("XScale.Maximum"=w6, "XScale.Minimum"=w5) -> ()  [unwired: 2 in, 2 out]
    }
  }
  n14 = call <vilib>:"Add State(s) to Queue__jki_lib_state_machine.vi"("State(s) in (\"\")"=w2) -> ("States Out"=w4:string)  [unwired: 14 in]
  n15 = while "Read Configed Ports SM" {
    shift-right: [w22] -> _
    shift-left: _ -> [w21]
    shift-right: [w24] -> _
    shift-left: _ -> [w19]
    shift-right: [w23] -> _
    shift-left: w4 -> [w25]
    tunnel: [w18] -> w3
    stop <- w18 stop-if-true
    n16 = call <vilib>:"Parse State Queue__jki_lib_state_machine.vi"("State Queue"=w25, "Error In (no error)"=w19) -> ("Remaining States"=w27:string, "Current State"=w28:string, "Arguments"=w26:string)  [unwired: 11 in]
    "Current State" <- w28
    n17 = call "E-Time.vi"() -> ("Elapsed Time (sec)"=w17:dbl)  [unwired: 9 in, 2 out]
    n18 = case shown="\"Write\"" w28 {
      selector: w28 -> [_ _ w79 _ _ _ _ _ _ _ _ w206 _ _ w256 _ _ _ _ _ _ _ _ _ _ _]
      tunnel: w27 -> [w35 w78 w83 w101 w107 w117 w121 w145 w156 w160 w185 w213 w236 w248 w261 w279 w290 w316 w321 w331 w335 w348 w472 w499 w567 w638]
      tunnel: w26 -> [_ _ _ _ _ _ _ _ _ _ _ _ _ _ w255 w274 w284 _ _ _ _ _ _ _ w535 _]
      tunnel: w21 -> [w33 w75 w81 w92 w104 w115 w118 _ w151 w157 w182 w211 w229 w245 w259 w277 w286 w313 w318 w328 w332 w355 w483 w493 w564 w635]
      tunnel: [w32 w76 w85 w98 errorcluster {"status"=FALSE, "code"=0, "source"=""} ("error out") w114 w119 w125 w152 w158 w183 w208 w233 w241 w250 w275 w287 w314 w319 w329 w333 w358 w484 w497 w565 w636] -> w24
      tunnel: w19 -> [w31 w76 w84 w98 w103 w114 w119 w126 w153 w158 w183 w209 w234 w241 w258 w276 w288 w314 w319 w329 w333 w358 w484 w497 w565 w636]
      tunnel: [w34 w77 w82 w100 w106 w116 w120 w144 w155 w159 w184 w212 w235 w247 w260 w278 w289 w315 w320 w330 w334 w359 w473 w498 w566 w637] -> w23
      tunnel: [_ _ _ _ _ TRUE _ _ _ _ _ _ _ _ _ _ _ _ _ _ _ _ _ _ _ _] -> w18
      tunnel: [w30 w75 w81 w99 w104 w115 w118 w143 w151 w157 w181 w211 w229 w244 w259 w277 w286 w313 w318 w328 w332 w354 w482 w492 w563 w635] -> w22
      tunnel: "Timeout" -> [w29 _ _ _ _ _ _ _ _ _ _ _ _ _ _ _ _ _ _ _ _ _ _ _ _ _]
      tunnel: w17 -> [_ _ _ _ _ _ _ _ _ _ _ _ _ _ _ _ _ _ _ _ _ _ _ _ _ _]
      frame "", "Idle" {
        # "executes when the state queue is empty"
        n19 = event shown="[2] \"Init\": Value Change" {
          selector: _ -> [_ _ _ _ _]
          dyn-events: _ -> [_ _ _ _ _]
          timeout: w29 -> [_ _ _ _ _]
          tunnel: w35 -> [w40 w43 w57 w68 w74]
          tunnel: [w39 w43 w57 w67 w73] -> w34
          tunnel: w33 -> [w37 w42 w53 w65 w71]
          tunnel: [w38 w41 w56 w66 w72] -> w32
          tunnel: w31 -> [w38 w41 w56 w66 w72]
          tunnel: [w37 w42 w53 w65 w71] -> w30
          event Timeout {
            n20 = event-data() -> ()  [unwired: 1 in, 1 out]
            n21 = call <vilib>:"Add State(s) to Queue__jki_lib_state_machine.vi"("State(s) in Front (\"\")"="Read\nGet Currents\nAdd Select Data\nCheck Power" ("State(s) in Front (\"\")"), "State(s) in (\"\")"=w40) -> ("States Out"=w39:string)  [unwired: 13 in]
          }
          event "Select Station": Value Change {
            n22 = event-data() -> ()  [unwired: 1 in, 6 out]
            n23 = local write "Command:Data"("" ("Command:Data")) -> ()
          }
          event "Init": Value Change {
            w50 = u8 128  # Tester Source Address
            w49 = u8 36  # Dryer Destination Address
            n24 = event-data() -> ()  [unwired: 1 in, 6 out]
            n25 = Unbundle By Name(w53) -> ("Com Array"=w55:u8[], "Label Com Array"=w54:string[][])
            n26 = for {
              tunnel: w54 -> [w63] mode=indexing
              tunnel: w55 -> [w58] mode=indexing
              tunnel: [w58] -> w52
              stop <- w60 stop-if-true
              n27 = local read "Select Station"() -> (w59:string)
              n28 = Index Array(array=w63, index=0) -> (element=w61:string)
              n29 = Equal?(x=w61, y=w59) -> (x = y?=w60:bool)
            }
            n30 = call "Com Chan Type Conversion.vi"("Com Chan"=w52) -> ("VISA resource name"=w48:refnum<visa-resource-name>)  [unwired: 11 in, 3 out]
            n31 = call "GEA2_ICP_Dryer_SM.vi"("ComPort"=w48, "Destination Address"=w49, "Source Address"=w50, "Mode"=GEA2_Dryer_Interface_Ctrl."Send WILT Startup CMDs") -> ("WriteOK"=→"Read_ACK":bool, "Error Out"=w47:errorcluster)  [unwired: 6 in, 4 out]
            n32 = call "GEA2_ICP_Dryer_SM.vi"("ComPort"=w48, "Destination Address"=w49, "Source Address"=w50, "Mode"=GEA2_Dryer_Interface_Ctrl."Send Continue CMD", "Error In"=w47) -> ()  [unwired: 5 in, 6 out]
          }
          event "Exit": Value Change {
            # "Exit Button Value Change (pressed) Event\n(this executes Macro: Exit to terminate the VI)"
            n33 = event-data() -> ()  [unwired: 1 in, 1 out]
            n34 = call <vilib>:"Add State(s) to Queue__jki_lib_state_machine.vi"("State(s) in Front (\"\")"="Macro: Exit", "State(s) in (\"\")"=w68) -> ("States Out"=w67:string)  [unwired: 13 in]
          }
          event Panel Close? {
            # "Discard the event because we'll close the front panel ourselves in Macro: Exit"
            # "Close Panel button (pressed) Event\n(this executes Macro: Exit to terminate the VI)"
            n35 = event-data() -> ()  [unwired: 1 in, 1 out]
            n36 = event-data("Discard?"=TRUE) -> ()  [unwired: 1 in, 1 out]
            n37 = call <vilib>:"Add State(s) to Queue__jki_lib_state_machine.vi"("State(s) in Front (\"\")"="Macro: Exit", "State(s) in (\"\")"=w74) -> ("States Out"=w73:string)  [unwired: 13 in]
          }
        }
      }
      frame "---------- Core ----------" {
        # "Do not put any code in this frame.\n(it is a separator no-op)"
        n38 = call <vilib>:"Add State(s) to Queue__jki_lib_state_machine.vi"("State(s) in (\"\")"=w78) -> ("States Out"=w77:string)  [unwired: 14 in]
      }
      frame Default {
        w88 = 42 items=["No error", "Argument error", "Memory is full", "Out of zone", "End of file", "File already open", "Generic file I/O error", "File not found", "File permission error", "Disk is full", "Duplicate path", "Too many files open", "System feature not enabled", "Resource file not found", "Cannot add resource", "Resource not found", "Image not found", "Image memory error", "Pen does not exist", "Config type invalid", "Config token not found", "Config parse error", "Config memory error", "Bad external code format", "Bad external code offset", "External code not present", "Null window", "Destroy window error", "Null menu", "Print aborted", "Bad print record", "Print driver error", "Windows error during printing", "Memory error during printing", "Print dialog error", "Generic print error", "Invalid device refnum", "Device not found", "Device parameter error", "Device unit error", "Cannot open device", "Device call aborted", "Generic error", "Cancelled by user", "Object ID too low", "Object ID too high", "Object not in heap", "Unknown heap", "Unknown object (invalid DefProc)", "Unknown object (DefProc not in table)", "Message out of range", "Invalid (null) method", "Unknown message", "Manager call not supported", "Bad address", "Network operation in progress", "Network operation timed out", "Connection is busy", "Network attribute not supported", "Network error", "Address in use", "System out of memory", "Connection aborted", "Connection refused", "Not connected", "Already connected", "Connection closed", "Initialization error (interapplication manager)", "Bad occurrence", "Wait on unbound occurrence handler", "Occurrence queue overflow", "Datalog type conflict", "Unused", "Unrecognized type (interapplication manager)", "Memory corrupt", "Failed to make temporary DLL", "Old CIN version", "Drag socket not found", "Failed to load drop-object", "Failed to register OLE object", "Failed to release OLE object", "Format specifier type mismatch", "Unknown format specifier", "Too few format specifiers", "Too many format specifiers", "Scan failed", "Newer CIN version", "Error converting to variant", "Runtime menu error", "Password tampered", "Variant attribute not found", "Incompatible variant data type", "Event data is not available", "Event Store is not present", "Occurrence is not found", "Event Queue is not created", "Event info is not available", "Refnum passed is NULL", "Error retrieving Class GUID", "Error retrieving CoClass GUID", "Error retrieving TypeLib GUID.", "Bad built application magic bytes.", "Specific driver is different from the specific driver associated with the Logical Name.", "There is no session opened to the class driver.", "Max Error", "MAX - Error with config objects", "MAX - Error loading configuration", "MAX - Group not supported"]
        # "Current State"
        # "Do not delete, rename, or modify this frame.\n(this is used to capture unhandled states and typos)"
        # "Handle mistyped state name (developer tool)"
        n39 = Format Into String(format string="Software Exception: Unhandled State \"%s\"." ("message"), error in=w84, w79) -> (resulting string=w87:string, error out=w86:errorcluster)  [unwired: 1 in]
        n40 = call <vilib>:"Error Cluster From Error Code.vi"("show call chain? (False)"=TRUE, "error in (no error)"=w86, "error message (\"\")"=w87, "error code (0)"=w88) -> ("error out"=w85:errorcluster)  [unwired: 5 in]
        n41 = call <vilib>:"Add State(s) to Queue__jki_lib_state_machine.vi"("State(s) in (\"\")"=w83) -> ("States Out"=w82:string)  [unwired: 14 in]
      }
      frame "Initialize Core Data" {
        # "Do not delete, rename, or modify this frame.\n(this is used to determine panel behavior on exit)"
        # "originally closed?"
        # "exe?"
        # "If panel starts closed or is an EXE, then close it when we exit"
        n42 = property class="VI"() -> ("Front Panel.Open"=w97:bool)  [unwired: 2 in, 2 out]
        n43 = property class="App"() -> ("App.Kind"=w96:T6)  [unwired: 2 in, 2 out]
        n44 = control-ref of="Current VI Reference"() -> (w90:refnum<vi>)
        n45 = Not(x=w97) -> (.not. x?=w94:bool)
        n46 = Equal?(x=w96, y=T6."Run Time System" ("Application:Kind")) -> (x = y?=w93:bool)
        n47 = Or(x=w94, y=w93) -> (x .or. y?=w91:bool)
        n48 = Bundle By Name(cluster=w92, "Core.Current VI Reference"=w90, "Core.Close Panel on Exit?"=w91) -> (w99:T8)
        n49 = call <vilib>:"Add State(s) to Queue__jki_lib_state_machine.vi"("State(s) in (\"\")"=w101) -> ("States Out"=w100:string)  [unwired: 14 in]
      }
      frame "Error Handler" {
        # "Unhandled Error -- Display it"
        # "Handle any errors here.\nYou can also output any states to clean-up after errors occur"
        # "Clear error"
        n50 = call <vilib>:"General Error Handler.vi"("error in (no error)"=w103) -> ()  [unwired: 10 in, 5 out]
        n51 = call <vilib>:"Add State(s) to Queue__jki_lib_state_machine.vi"("State(s) in Front (\"\")"="/* Post Error States", "State(s) in (\"\")"=w107) -> ("States Out"=w106:string)  [unwired: 13 in]
      }
      frame "Exit" {
        # "Do not put any code in this frame.\n(No errors that occur here will be handled.)"
        n52 = local read "Filename Currents"() -> (w108:path)
        n53 = local read "Low Lim 2"() -> (w110:dbl[])
        n54 = local read "Low Lim"() -> (w111:dbl[])
        n55 = local read "Up Lim"() -> (w112:dbl[])
        n56 = call "RW Current Limits.vi"("Write?"=TRUE, "Low Lim 2"=w110, "Low Lim"=w111, "Up Lim"=w112, "file path (dialog if empty)"=w108) -> ()  [unwired: 4 in, 3 out]
        n57 = call <vilib>:"Add State(s) to Queue__jki_lib_state_machine.vi"("State(s) in (\"\")"=w117) -> ("States Out"=w116:string)  [unwired: 14 in]
      }
      frame "---------- Data ----------" {
        # "Do not put any code in this frame.\n(It is a separator no-op. You can make a copy of this frame to create a new Data frame)"
        n58 = call <vilib>:"Add State(s) to Queue__jki_lib_state_machine.vi"("State(s) in (\"\")"=w121) -> ("States Out"=w120:string)  [unwired: 14 in]
      }
      frame "Data: Initialize" {
        w129 = 1 items=["one channel for each line", "one channel for all lines"] ("line grouping")
        w132 = ""  # Last Hour
        w134 = string[][] []  # Data to Save
        w137 = u8[] []  # Com Array
        w142 = T9 {"Current VI Reference"=refnum, "Close Panel on Exit?"=FALSE}  # Core
        # "Initialize the shift-register data, here.\n(data names are defined by what you wire into the bundle function)"
        n59 = stacked-sequence {
          frame #0 {
            w146 = FALSE ("A Alarm")
            n60 = local write "A Alarm"(w146) -> ()
            n61 = local write "B Alarm"(w146) -> ()
            n62 = local write "C Alarm"(w146) -> ()
            n63 = local write "D Alarm"(w146) -> ()
            n64 = local write "Ready"(w146) -> ()
          }
          frame #1 {
            w147 = string[][] []  # Data to Save
            n65 = local write "D Array"(w147) -> ()
            n66 = local write "C Array"(w147) -> ()
            n67 = local write "A Array"(w147) -> ()
            n68 = local write "B Array"(w147) -> ()
          }
          frame #2 {
            w148 = dbl[] [] ("D Data")
            n69 = local write "A Data"(w148) -> ()
            n70 = local write "C Data"(w148) -> ()
            n71 = local write "D Data"(w148) -> ()
            n72 = local write "B Data"(w148) -> ()
            n73 = local write "D Data 2"(w148) -> ()
            n74 = local write "C Data 2"(w148) -> ()
            n75 = local write "A Data 2"(w148) -> ()
            n76 = local write "B Data 2"(w148) -> ()
          }
        }
        n77 = call "Rising Edge Latch.vi"("Reset"=TRUE) -> ()  [unwired: 10 in, 1 out]
        n78 = call "Read From Spreadsheet File (string) with Prompt.vi"("delimiter (\\t)"="," ("delimiter (\\t)"), "prompt"="Choose config file to read.", "file path (dialog if empty)"="Config File") -> ("all rows"=w140:string[][])  [unwired: 4 in, 4 out]
        n79 = flat-sequence {
          tunnel: w140 -> [w149]
          tunnel: [w150] -> w139
          frame #0 {
            "Label Com Array" <- w149
          }
          frame #1 {
            n80 = local read "Label Com Array"() -> (w150:string[][])
          }
        }
        n81 = call "IP and Computer Name.vi"() -> ("Computer Name"=w130:string)  [unwired: 10 in, 1 out]
        "Computer Name" <- w130
        n82 = local write "Command:Data"(w132) -> ()
        n83 = call-poly <vilib>:"DAQmx Create Virtual Channel.vi"("lines"="Power Port", "line grouping"=w129, "error in"=w126) -> ("task out"=w127:refnum<k21>, "error out"=w128:errorcluster)  [unwired: 11 in]
        n84 = call <vilib>:"DAQmx Start Task.vi"("task/channels in"=w127, "error in"=w128) -> ("task out"=w123:refnum<k21>, "error out"=w125:errorcluster)  [unwired: 12 in]
        n85 = call <vilib>:"Add State(s) to Queue__jki_lib_state_machine.vi"("State(s) in (\"\")"=w145) -> ("States Out"=w144:string)  [unwired: 14 in]
        n86 = Bundle("Core"=w142, "Data to Save"=w134, "Label Com Array"=w139, "UI Array"="UI Array", "Com Array"=w137, "Save File Path"="Save File Path", "Last Hour"=w132, "Computer Name"=w130, "task out"=w123, "Power"="Power") -> (w143:T8)  [unwired: 1 in]
      }
      frame "Data: Cleanup" {
        # "Cleanup any data and references, here.\n(this is called automatically, by the Macro: Exit)"
        n87 = Unbundle By Name(w151) -> ("Core.Current VI Reference"=w154:refnum<vi>)
        n88 = Close Reference(reference=w154, error in (no error)=w153) -> (error out=w152:errorcluster)
        n89 = call <vilib>:"Add State(s) to Queue__jki_lib_state_machine.vi"("State(s) in (\"\")"=w156) -> ("States Out"=w155:string)  [unwired: 14 in]
      }
      frame "---------- UI ----------" {
        # "Do not put any code in this frame.\n(It is a separator no-op. You can make a copy of this frame to create a new UI frame)"
        n90 = call <vilib>:"Add State(s) to Queue__jki_lib_state_machine.vi"("State(s) in (\"\")"=w160) -> ("States Out"=w159:string)  [unwired: 14 in]
      }
      frame "UI: Initialize" {
        # "Initialize the User Interface, here.\n(this is called automatically, by the Macro: Init)"
        n91 = local read "Cycle Count Path"() -> (w162:path)
        n92 = Unbundle By Name(w182) -> ("Label Com Array"=w171:string[][])
        n93 = call <vilib>:"Check if File or Folder Exists.vi"("path"=w162) -> ("file or folder exists?"=w161:bool)  [unwired: 8 in, 2 out]
        n94 = Transpose 2D Array(2D array=w171) -> (transposed array=w172:string[][])
        n95 = case shown="False" w161 {
          tunnel: [dbl[][] [[0.0, 0.0], [0.0, 0.0], [0.0, 0.0], [0.0, 0.0]] ("all rows") w189] -> w167
          tunnel: w162 -> [_ w187]
          frame False {
          }
          frame True {
            n96 = call-poly <vilib>:"Read From Spreadsheet File.vi"("delimiter (\\t)"="," ("element"), "file path (dialog if empty)"=w187) -> ("all rows"=w189:dbl[][])  [unwired: 5 in, 4 out]
          }
        }
        n97 = call "Array-Get 1D Row fr 2D str.vi"("all rows"=w172, "row index"=0) -> ("row"=w169:string[])  [unwired: 13 in]
        n98 = property on="Select Station" class="CmbBox"("Strings[]"=w169) -> ()  [unwired: 2 in, 2 out]
        n99 = Index Array(array=w167, index (col)=1 ("disabled index (col)")) -> (element=w165:dbl[])  [unwired: 1 in]
        n100 = Delete From Array(array=w165, length=4) -> (deleted portion=w163:dbl[])  [unwired: 1 in, 1 out]
        n101 = for {
          tunnel: w171 -> [w204] mode=indexing
          tunnel: [w193] -> w180 mode=indexing
          tunnel: [w198] -> w174 mode=indexing
          tunnel: [w196] -> w179
          tunnel: [w192] -> w168 mode=indexing
          tunnel: w163 -> [w190] mode=indexing
          i -> [w197]
          (unwired) 1 ("index")
          n102 = Index Array(array=w204, index #1=0 ("index"), index #2=1 ("index")) -> (element #1=w200:string, element #2=w199:string)
          n103 = Decimal String To Number(string=w199) -> (number=w195:i32)  [unwired: 2 in, 1 out]
          n104 = To Unsigned Long Integer(number=w190) -> (unsigned 32bit integer=w191:u32)
          n105 = Bundle By Name(cluster=T4 {"Label"="M1", "Color"=0, "Last Read Status"=enum."Err", "Command:Data"="", "Err Count"=0, "Cycle Count"=0} ("Location:IND,Status,Message,No Com Count, Cycle Count"), "Label"=w200, "Cycle Count"=w191) -> (w198:T4)
          n106 = To Unsigned Byte Integer(number=w195) -> (unsigned 8bit integer=w193:u8)
          n107 = Increment(x=w197) -> (x+1=w196:i32)
          n108 = Bundle By Name(cluster=T2 {"Color"=0, "Last Read Status"=enum."Err", "Command:Data"="", "Com Port"=0, "Time(S)"=0.0, "Err Count"=0} ("Dryer Status Serial Data In"), "Com Port"=w193) -> (w192:T2)
        }
        n109 = call <vilib>:"Add State(s) to Queue__jki_lib_state_machine.vi"("State(s) in (\"\")"=w185) -> ("States Out"=w184:string)  [unwired: 14 in]
        n110 = local write "Status Array Out"(w168) -> ()
        n111 = local write "UI Array"(w174) -> ()
        n112 = Bundle By Name(cluster=w182, "UI Array"=w174, "Com Array"=w180) -> (w181:T8)
        n113 = In Range and Coerce(upper limit=20, x=w179, lower limit=1) -> (coerced(x)=w176:i32, In Range?=w175:bool)
        n114 = Not(x=w175) -> (.not. x?=w173:bool)
        n115 = property on="UI Array" class="Arr (strict)"("Number of Rows"=w176, "VertScroll"=w173) -> ()  [unwired: 2 in, 2 out]
      }
      frame "Init Com Ports" {
        # "Initialize the User Interface, here.\n(this is called automatically, by the Macro: Init)"
        n116 = Unbundle By Name(w211) -> ("Com Array"=w210:u8[])
        n117 = for {
          tunnel: w210 -> [w224] mode=indexing
          shift-right: [w221] -> w208
          shift-left: w209 -> [w225]
          tunnel: [w222] -> w207
          stop <- w221 stop-if-true
          n118 = call "Com Chan Type Conversion.vi"("Com Chan"=w224) -> ("VISA resource name"=w222:refnum<visa-resource-name>)  [unwired: 11 in, 3 out]
          n119 = call "GEA2_ICP_Dryer_SM.vi"("ComPort"=w222, "Mode"=GEA2_Dryer_Interface_Ctrl."Init Com Port", "Error In"=w225) -> ("Error Out"=w223:errorcluster)  [unwired: 7 in, 5 out]
          n120 = call "GEA2_ICP_Dryer_SM.vi"("ComPort"=w222, "Mode"=GEA2_Dryer_Interface_Ctrl."Send WILT Startup CMDs", "Error In"=w223) -> ("Error Out"=w221:errorcluster)  [unwired: 7 in, 5 out]
        }
        n121 = case shown="Error" w208 {
          tunnel: w207 -> [_ w217]
          tunnel: w206 -> [_ w216]
          tunnel: [_ "Exit" ("State(s) in Front (\"\")")] -> w205
          frame No Error {
          }
          frame Error {
            n122 = call "Com Chan Type Conversion.vi"("Com Chan In"=w217) -> ("Com Text 2"=w214:string)  [unwired: 11 in, 3 out]
            n123 = Concatenate Strings(w216, w214) -> (w218:string)
            n124 = One Button Dialog(message=w218) -> ()  [unwired: 1 in, 1 out]
          }
        }
        n125 = call <vilib>:"Add State(s) to Queue__jki_lib_state_machine.vi"("State(s) in Front (\"\")"=w205, "State(s) in (\"\")"=w213) -> ("States Out"=w212:string)  [unwired: 13 in]
      }
      frame "Init Power" {
        w232 = TRUE  # Valves Off
        # "Initialize the User Interface, here.\n(this is called automatically, by the Macro: Init)"
        n126 = Unbundle By Name(w229) -> ("task out"=w228:refnum<k21>, "Power"=w226:bool[])
        n127 = Build Array(w232, w232, w232, w232) -> (w231:bool[])
        n128 = Build Array (concatenate)(w231, w226) -> (w227:bool[])
        n129 = Boolean Array To Number(Boolean array=w227) -> (number=w230:u32)
        n130 = call-poly <vilib>:"DAQmx Write.vi"("task/channels in"=w228, "data"=w230, "error in"=w234) -> ("error out"=w233:errorcluster)  [unwired: 10 in, 2 out]
        n131 = call <vilib>:"Add State(s) to Queue__jki_lib_state_machine.vi"("State(s) in (\"\")"=w236) -> ("States Out"=w235:string)  [unwired: 14 in]
      }
      frame "Init Labels" {
        # "Initialize the User Interface, here.\n(this is called automatically, by the Macro: Init)"
        n132 = Unbundle By Name(w245) -> ("Label Com Array"=w246:string[][])
        n133 = call "Panel SS Station Labels.vi"("Label Com Array"=w246) -> ("Array Out"=w237:string[][])  [unwired: 10 in]
        n134 = local read "Config File"() -> (w243:path)
        n135 = Transpose 2D Array(2D array=w237) -> (transposed array=w240:string[][])
        n136 = Bundle By Name(cluster=w245, "Label Com Array"=w237) -> (w244:T8)
        n137 = call "Array-Get 1D Row fr 2D str.vi"("all rows"=w240, "row index"=0) -> ("row"=w238:string[])  [unwired: 13 in]
        n138 = call-poly <vilib>:"Write To Spreadsheet File.vi"("delimiter (\\t)"="," ("delimiter (\\t)"), "2D data"=w237, "file path (dialog if empty)"=w243) -> ()  [unwired: 5 in, 1 out]
        n139 = property on="Select Station" class="CmbBox"("Strings[]"=w238) -> ()  [unwired: 2 in, 2 out]
        n140 = local write "Label Com Array"(w237) -> ()
        n141 = call <vilib>:"Add State(s) to Queue__jki_lib_state_machine.vi"("State(s) in (\"\")"=w248) -> ("States Out"=w247:string)  [unwired: 14 in]
      }
      frame "Send Restart" {
        # "send the restart command"
        n142 = case shown="\"D\"" w255 {
          tunnel: [2 ("index") 3 ("index") 0 ("index") 1 ("index")] -> w253
          frame "C", Default {
          }
          frame "D" {
          }
          frame "A" {
          }
          frame "B" {
          }
        }
        n143 = Unbundle By Name(w259) -> ("Com Array"=w254:u8[])
        n144 = Index Array(array=w254, index=w253) -> (element=w252:u8)
        n145 = call "Com Chan Type Conversion.vi"("Com Chan"=w252) -> ("VISA resource name"=w257:refnum<visa-resource-name>)  [unwired: 11 in, 3 out]
        n146 = call "GEA2_ICP_Dryer_SM.vi"("ComPort"=w257, "Mode"=GEA2_Dryer_Interface_Ctrl."Send Continue CMD", "Error In"=w258) -> ("Error Out"=w251:errorcluster)  [unwired: 7 in, 5 out]
        n147 = case shown="No Error" w251 {
          selector: w251 -> [w266 w268]
          tunnel: w257 -> [_ w271]
          tunnel: w256 -> [_ w270]
          tunnel: [w266 w267] -> w250
          frame No Error {
          }
          frame Error {
            n148 = call "Com Chan Type Conversion.vi"("Com Chan In"=w271) -> ("Com Text"=w272:string)  [unwired: 11 in, 3 out]
            n149 = call "Counter.vi"() -> ("Count"=→"Restart Err Count":dbl)  [unwired: 11 in]
            n150 = call <vilib>:"Clear Errors.vi"("error in (no error)"=w268) -> ("error out"=w267:errorcluster)  [unwired: 6 in]
            n151 = Concatenate Strings(w270, w272) -> (→"Com Er Mess":string)
          }
        }
        n152 = call <vilib>:"Add State(s) to Queue__jki_lib_state_machine.vi"("State(s) in (\"\")"=w261) -> ("States Out"=w260:string)  [unwired: 14 in]
      }
      frame "UI: Cursor Set" {
        # "Argument"
        # "Set and Unset Cursor Busy.\n(Usage: \"UI: Cursor Set >> Busy|Idle\")"
        n153 = case shown="\"Idle\", Default" w274 {
          tunnel: w276 -> [w281 w283]
          tunnel: [w280 w282] -> w275
          frame "Idle", Default {
            n154 = call <vilib>:"Unset Busy.vi"("error in (no error)"=w281) -> ("error out"=w280:errorcluster)  [unwired: 10 in]
          }
          frame "Busy" {
            n155 = call <vilib>:"Set Busy.vi"("error in (no error)"=w283) -> ("error out"=w282:errorcluster)  [unwired: 9 in, 1 out]
          }
        }
        n156 = call <vilib>:"Add State(s) to Queue__jki_lib_state_machine.vi"("State(s) in (\"\")"=w279) -> ("States Out"=w278:string)  [unwired: 14 in]
      }
      frame "UI: Front Panel State" {
        # "Argument"
        # "Set Front Panel Open or Closed\n(Usage: \"UI: Front Panel State >> Open|Close\")"
        n157 = Unbundle By Name(w286) -> ("Core.Current VI Reference"=w285:refnum<vi>)
        n158 = case shown="\"Open\", Default" w284 {
          tunnel: w288 -> [w294 w307]
          tunnel: [w296 w308] -> w287
          tunnel: w285 -> [w295 w305]
          frame "Open", Default {
            n159 = property class="VI"(reference=w295, error in=w294) -> (reference out=w292:refnum<vi>, error out=w293:errorcluster, "Front Panel.Open"=w291:bool)
            n160 = case shown="False" w291 {
              tunnel: [w299 w302] -> w296
              tunnel: w293 -> [w298 w302]
              tunnel: w292 -> [w297 _]
              frame False {
                n161 = invoke class="VI" method="FP.Open"(reference=w297, error in=w298, "Activate"=TRUE, "State"=T7."Standard") -> (error out=w299:errorcluster)  [unwired: 1 in, 4 out]
              }
              frame True {
              }
            }
          }
          frame "Close" {
            n162 = property class="VI"(reference=w305, error in=w307) -> (reference out=w304:refnum<vi>, error out=w306:errorcluster, "Front Panel.Open"=w303:bool)
            n163 = case shown="True" w303 {
              tunnel: [w309 w312] -> w308
              tunnel: w306 -> [w309 w311]
              tunnel: w304 -> [_ w310]
              frame False {
              }
              frame True {
                n164 = invoke class="VI" method="FP.Close"(reference=w310, error in=w311) -> (error out=w312:errorcluster)  [unwired: 1 in, 2 out]
              }
            }
          }
        }
        n165 = call <vilib>:"Add State(s) to Queue__jki_lib_state_machine.vi"("State(s) in (\"\")"=w290) -> ("States Out"=w289:string)  [unwired: 14 in]
      }
      frame "---------- Macro ----------" {
        # "Do not put any code in this frame.\n(It is a separator no-op. You can make a copy of this frame to create a new Macro frame)"
        n166 = call <vilib>:"Add State(s) to Queue__jki_lib_state_machine.vi"("State(s) in (\"\")"=w316) -> ("States Out"=w315:string)  [unwired: 14 in]
      }
      frame "Macro: Initialize" {
        w317 = "Data: Initialize\nInitialize Core Data\nUI: Initialize\nUI: Front Panel State >> Open\nInit Com Ports"  # Data: Initialize Initialize Core Data UI: Initialize UI: Front Panel State >> Open Init Com Ports
        # "Initialization Macro\n(This is called once, when the VI starts)"
        n167 = call <vilib>:"Add State(s) to Queue__jki_lib_state_machine.vi"("State(s) in Front (\"\")"=w317, "State(s) in (\"\")"=w321) -> ("States Out"=w320:string)  [unwired: 13 in]
      }
      frame "Macro: Exit" {
        # "Exit Macro\n(This is called once, when the VI exits)"
        n168 = Unbundle By Name(w328) -> ("Core.Close Panel on Exit?"=w327:bool)
        n169 = Select(t="UI: Front Panel State >> Close", s=w327, f="") -> (s? t:f=w324:string)
        n170 = call <vilib>:"Add State(s) to Queue__jki_lib_state_machine.vi"("State(s) in (\"\")"=w324, "State(s) at Back (\"\")"="Data: Cleanup\nExit") -> ("States Out"=w322:string)  [unwired: 13 in]
        n171 = call <vilib>:"Add State(s) to Queue__jki_lib_state_machine.vi"("State(s) in Front (\"\")"=w322, "State(s) in (\"\")"=w331) -> ("States Out"=w330:string)  [unwired: 13 in]
      }
      frame "---------- New Category ----------" {
        # "Template Separator\n(You can make a copy of, or modify, this frame)"
        n172 = call <vilib>:"Add State(s) to Queue__jki_lib_state_machine.vi"("State(s) in (\"\")"=w335) -> ("States Out"=w334:string)  [unwired: 14 in]
      }
      frame "Get Currents" {
        n173 = Unbundle By Name(w355) -> ("UI Array"=w356:T4[])
        n174 = call "Rising Edge Latch.vi"() -> ("Rising Edge Out"=w339:bool[])  [unwired: 11 in]
        "Rising Edge Out" <- w339
        n175 = local read "Max Len"() -> (w336:i32)
        n176 = stacked-sequence {
          tunnel: "Up Lim" -> [w390 w405 w420 w435]
          tunnel: "Low Lim" -> [w389 w404 w419 w434]
          tunnel: w336 -> [w386 w401 w417 w431]
          tunnel: [w382 _ _ _] -> w347
          tunnel: [_ w398 _ _] -> w346
          tunnel: [_ _ w414 _] -> w345
          tunnel: [_ _ _ w430] -> w351
          tunnel: "Low Lim 2" -> [w385 w400 w415 w429]
          frame #0 {
            n177 = call "SS Current Test.vi"("Lower Limit 2"=w385, "Lower Limit"=w389, "Y 2"="A Data 2", "Y"="A Data", "Upper Limit"=w390) -> ("Out of Bounds"=w383:bool, "Waveform Chart"=→"Station A: L1 Current":waveform(dbl)[])  [unwired: 5 in]
            "A Alarm" <- w383
            n178 = Array Size(array="A Data") -> (size(s)=w387:i32)
            n179 = Equal?(x=w387, y=w386) -> (x = y?=w384:bool)
            n180 = case shown="True" w384 {
              tunnel: [_ w394] -> w382
              tunnel: w383 -> [_ w393]
              frame False {
              }
              frame True {
                n181 = case shown="True" w393 {
                  tunnel: ["Write >> A" "Send Restart >> A"] -> w394
                  frame True {
                  }
                  frame False {
                  }
                }
              }
            }
          }
          frame #1 {
            n182 = call "SS Current Test.vi"("Lower Limit 2"=w400, "Lower Limit"=w404, "Y 2"="B Data 2", "Y"="B Data", "Upper Limit"=w405) -> ("Out of Bounds"=w397:bool, "Waveform Chart"=→"Station B: L1 Current":waveform(dbl)[])  [unwired: 5 in]
            "B Alarm" <- w397
            n183 = Array Size(array="B Data") -> (size(s)=w402:i32)
            n184 = Equal?(x=w401, y=w402) -> (x = y?=w399:bool)
            n185 = case shown="True" w399 {
              tunnel: [_ w409] -> w398
              tunnel: w397 -> [_ w408]
              frame False {
              }
              frame True {
                n186 = case shown="True" w408 {
                  tunnel: ["Write >> B" "Send Restart >> B"] -> w409
                  frame True {
                  }
                  frame False {
                  }
                }
              }
            }
          }
          frame #2 {
            n187 = call "SS Current Test.vi"("Lower Limit 2"=w415, "Lower Limit"=w419, "Y 2"="C Data 2", "Y"="C Data", "Upper Limit"=w420) -> ("Out of Bounds"=w412:bool, "Waveform Chart"=→"Station C: L1 Current":waveform(dbl)[])  [unwired: 5 in]
            "C Alarm" <- w412
            n188 = Array Size(array="C Data") -> (size(s)=w418:i32)
            n189 = Equal?(x=w417, y=w418) -> (x = y?=w413:bool)
            n190 = case shown="True" w413 {
              tunnel: [_ w424] -> w414
              tunnel: w412 -> [_ w423]
              frame False {
              }
              frame True {
                n191 = case shown="False" w423 {
                  tunnel: ["Write >> C" "Send Restart >> C"] -> w424
                  frame True {
                  }
                  frame False {
                  }
                }
              }
            }
          }
          frame #3 {
            n192 = call "SS Current Test.vi"("Lower Limit 2"=w429, "Lower Limit"=w434, "Y 2"="D Data 2", "Y"="D Data", "Upper Limit"=w435) -> ("Out of Bounds"=w427:bool, "Waveform Chart"=→"Station D: L1 Current":waveform(dbl)[])  [unwired: 5 in]
            "D Alarm" <- w427
            n193 = Array Size(array="D Data") -> (size(s)=w433:i32)
            n194 = Equal?(x=w431, y=w433) -> (x = y?=w428:bool)
            n195 = case shown="True" w428 {
              tunnel: [_ w439] -> w430
              tunnel: w427 -> [_ w438]
              frame False {
              }
              frame True {
                n196 = case shown="False" w438 {
                  tunnel: ["Write >> D" "Send Restart >> D"] -> w439
                  frame True {
                  }
                  frame False {
                  }
                }
              }
            }
          }
        }
        n197 = for {
          tunnel: w339 -> [w381] mode=indexing
          tunnel: w356 -> [w380] mode=indexing
          tunnel: [w377] -> w342 mode=indexing
          tunnel: [TRUE] -> w357
          tunnel: [w373] -> w340 mode=indexing
          tunnel: [w369] -> w341 mode=indexing
          n198 = Boolean To (0,1)(Boolean=w381) -> (0, 1=w378:i16)
          n199 = Unbundle By Name(w380) -> ("Label"=w370:string, "Cycle Count"=w379:u32)
          n200 = To Unsigned Long Integer(number=w378) -> (unsigned 32bit integer=w368:u32)
          n201 = Add(x=w379, y=w368) -> (x+y=w372:u32)
          n202 = Quotient & Remainder(x=w372, y="Cycle Save Multiple") -> (x-y*floor(x/y)=w374:u32)  [unwired: 1 out]
          n203 = Bundle By Name(cluster=w380, "Cycle Count"=w372) -> (w377:T4)
          n204 = Equal To 0?(x=w374) -> (x = 0?=w373:bool)
          n205 = Number To Decimal String(number=w372) -> (decimal integer string=w371:string)  [unwired: 1 in]
          n206 = Build Array(w370, w371) -> (w369:string[])
        }
        n207 = And(x=w340, y=w339) -> (x .and. y?=w338:bool[])
        n208 = call "Rising Edge Latch.vi"("Reset"=w357) -> ()  [unwired: 10 in, 1 out]
        n209 = call <vilib>:"Add State(s) to Queue__jki_lib_state_machine.vi"("State(s) in Front (\"\")"=w347, "State(s) in (\"\")"=w348) -> ("States Out"=w349:string)  [unwired: 13 in]
        n210 = Or Array Elements(Boolean array=w338) -> (logical OR=w337:bool)
        n211 = local write "UI Array"(w342) -> ()
        n212 = case shown="True" w337 {
          tunnel: w341 -> [_ w363]
          frame False {
          }
          frame True {
            n213 = call "Log String to Spreadsheet.vi"("String"="Count Log", "FileName"="Cycle Count Path") -> ("error out"=w360:errorcluster)  [unwired: 9 in]
            n214 = flat-sequence {
              tunnel: w363 -> [w367]
              tunnel: "Cycle Count Path" -> [w365]
              tunnel: w360 -> [_]
              frame #0 {
                n215 = call-poly <vilib>:"Write To Spreadsheet File.vi"("delimiter (\\t)"="," ("delimiter (\\t)"), "append to file? (new file:F)"=TRUE, "2D data"=w367, "file path (dialog if empty)"=w365) -> ()  [unwired: 4 in, 1 out]
              }
            }
          }
        }
        n216 = call <vilib>:"Add State(s) to Queue__jki_lib_state_machine.vi"("State(s) in Front (\"\")"=w346, "State(s) in (\"\")"=w349) -> ("States Out"=w350:string)  [unwired: 13 in]
        n217 = call <vilib>:"Add State(s) to Queue__jki_lib_state_machine.vi"("State(s) in Front (\"\")"=w345, "State(s) in (\"\")"=w350) -> ("States Out"=w344:string)  [unwired: 13 in]
        n218 = Bundle By Name(cluster=w355, "UI Array"=w342) -> (w354:T8)
        n219 = call <vilib>:"Add State(s) to Queue__jki_lib_state_machine.vi"("State(s) in Front (\"\")"=w351, "State(s) in (\"\")"=w344) -> ("States Out"=w359:string)  [unwired: 13 in]
      }
      frame "Check Power" {
        # "Last read current."
        # "True means turn power off."
        # "Your code here.\n(You can make a copy of, or modify, this frame)"
        n220 = global read "Globals SS.vi" "D L1 index"() -> (w443:i32)
        n221 = global read "Globals SS.vi" "C L1 index"() -> (w444:i32)
        n222 = global read "Globals SS.vi" "A L1 Index"() -> (w446:i32)
        n223 = global read "Globals SS.vi" "B L1 index"() -> (w445:i32)
        n224 = local read "Max Len"() -> (w442:i32)
        n225 = local read "D Data"() -> (w454:dbl[])
        n226 = local read "A Data"() -> (w461:dbl[])
        n227 = local read "B Data"() -> (w457:dbl[])
        n228 = local read "C Data"() -> (w456:dbl[])
        n229 = Array Size(array=w454) -> (size(s)=w455:i32)
        n230 = Array Size(array=w461) -> (size(s)=w460:i32)
        n231 = Array Size(array=w457) -> (size(s)=w458:i32)
        n232 = Array Size(array=w456) -> (size(s)=w453:i32)
        n233 = local read "Currents"() -> (w481:dbl[])
        n234 = local read "A Alarm"() -> (w466:bool)
        n235 = local read "B Alarm"() -> (w467:bool)
        n236 = local read "C Alarm"() -> (w468:bool)
        n237 = local read "D Alarm"() -> (w469:bool)
        n238 = Greater Or Equal?(x=w453, y=w442) -> (x >= y?=w450:bool)
        n239 = Greater Or Equal?(x=w455, y=w442) -> (x >= y?=w449:bool)
        n240 = Greater Or Equal?(x=w460, y=w442) -> (x >= y?=w452:bool)
        n241 = Greater Or Equal?(x=w458, y=w442) -> (x >= y?=w451:bool)
        n242 = local read "Off On Threshold"() -> (w447:dbl)
        n243 = Index Array(array=w481, index #1=w446, index #2=w445, index #3=w444, index #4=w443) -> (element #1=w480:dbl, element #2=w479:dbl, element #3=w478:dbl, element #4=w477:dbl)
        n244 = Bundle(w452, w451, w450, w449) -> (w459:cluster{bool, bool, bool, bool})  [unwired: 1 in]
        n245 = Bundle("A Alarm"=w466, "B Alarm"=w467, "C Alarm"=w468, "D Alarm"=w469) -> (w465:T10)  [unwired: 1 in]
        n246 = Bundle("Waveform"=w480, "Waveform"=w479, "Waveform"=w478, "Waveform"=w477) -> (w476:T11)  [unwired: 1 in]
        n247 = Cluster To Array(cluster=w459) -> (array=w448:bool[])
        n248 = Cluster To Array(cluster=w476) -> (array=w475:dbl[])
        n249 = Cluster To Array(cluster=w465) -> (array=w464:bool[])
        n250 = Greater?(x=w475, y=w447) -> (0:w463:bool[])
        n251 = Compound Arithmetic op=AND(w464, w463, w448) -> (w462:bool[])
        n252 = Not(x=w462) -> (.not. x?=w474:bool[])
        n253 = Or Array Elements(Boolean array=w474) -> (logical OR=w471:bool)
        n254 = case shown="True" w471 {
          tunnel: [_ "Init Power" ("State(s) in Front (\"\")")] -> w470
          frame False {
          }
          frame True {
          }
        }
        n255 = call <vilib>:"Add State(s) to Queue__jki_lib_state_machine.vi"("State(s) in Front (\"\")"=w470, "State(s) in (\"\")"=w472) -> ("States Out"=w473:string)  [unwired: 13 in]
        n256 = Bundle By Name(cluster=w483, "Power"=w462) -> (w482:T8)
      }
      frame "Read" {
        # "read all the com array ports, and update the gui"
        n257 = call "Counter.vi"() -> ("Count"=→"Read Serial Count":dbl)  [unwired: 11 in]
        n258 = flat-sequence {
          tunnel: [w500] -> w486
          frame #0 {
            n259 = local read "Status Array Out"() -> (w500:T2[])
            n260 = local write "Reading"(TRUE ("Reading")) -> ()
          }
        }
        n261 = Unbundle By Name(w493) -> ("Label Com Array"=w490:string[][], "Com Array"=w496:u8[], "UI Array"=w494:T4[])
        n262 = call "Read All Dryers.vi"("Com Array"=w496, "Status Array In"=w486) -> ("Log Coms Array"=w489:string[], "Status Array Out"=w495:T2[], "Data Present"=w491:bool[])  [unwired: 10 in, 1 out]
        "Status Array Out" <- w495
        "Log Coms Array" <- w489
        n263 = for {
          tunnel: w495 -> [w518] mode=indexing
          tunnel: w494 -> [w517] mode=indexing
          tunnel: [w513] -> w488 mode=indexing
          tunnel: w491 -> [w509] mode=indexing
          tunnel: w490 -> [w512] mode=indexing
          tunnel: w489 -> [w510] mode=indexing
          i -> [w507]
          n264 = Index Array(array=w512, index=0) -> (element=w506:string)
          n265 = Unbundle By Name(w518) -> ("Color"=w516:u32, "Last Read Status"=w515:T3, "Command:Data"=w514:string, "Err Count"=w508:u32)
          n266 = case shown="True" w509 {
            tunnel: w506 -> [_ w534]
            tunnel: w510 -> [_ w532]
            tunnel: [_ w531] -> w505
            frame False {
            }
            frame True {
              n267 = Concatenate Strings(w534, "," ("string"), w532) -> (w531:string)
            }
          }
          n268 = case shown="0, Default" w507 {
            tunnel: w505 -> [w519 w522 w525 w528]
            frame 0, Default {
              n269 = local read "A Array"() -> (w520:string[][])
              n270 = call "Array - Insert on Bottom.vi"("New String"=w519, "appended array"=w520) -> ("output array"=→"A Array":string[][])  [unwired: 9 in]
            }
            frame 1 {
              n271 = local read "B Array"() -> (w523:string[][])
              n272 = call "Array - Insert on Bottom.vi"("New String"=w522, "appended array"=w523) -> ("output array"=→"B Array":string[][])  [unwired: 9 in]
            }
            frame 2 {
              n273 = local read "C Array"() -> (w526:string[][])
              n274 = call "Array - Insert on Bottom.vi"("New String"=w525, "appended array"=w526) -> ("output array"=→"C Array":string[][])  [unwired: 9 in]
            }
            frame 3 {
              n275 = local read "D Array"() -> (w529:string[][])
              n276 = call "Array - Insert on Bottom.vi"("New String"=w528, "appended array"=w529) -> ("output array"=→"D Array":string[][])  [unwired: 9 in]
            }
          }
          n277 = Bundle By Name(cluster=w517, "Color"=w516, "Last Read Status"=w515, "Command:Data"=w514, "Err Count"=w508) -> (w513:T4)
        }
        n278 = Bundle By Name(cluster=w493, "UI Array"=w488) -> (w492:T8)
        n279 = flat-sequence {
          tunnel: w488 -> [w504]
          frame #0 {
            n280 = local write "UI Array"(w504) -> ()
            "Reading" <- FALSE ("Reading")
            "Ready" <- TRUE ("Reading")
          }
        }
        n281 = call <vilib>:"Add State(s) to Queue__jki_lib_state_machine.vi"("State(s) in (\"\")"=w499) -> ("States Out"=w498:string)  [unwired: 14 in]
      }
      frame "Write" {
        w536 = "_" ("string")
        # "SS"
        # "Writes the data file."
        n282 = Unbundle By Name(w564) -> ("Save File Path"=w540:path, "Label Com Array"=w550:string[][], "Last Hour"=w558:string, "Computer Name"=w551:string)
        n283 = case shown="\"D\"" w535 {
          tunnel: w550 -> [w575 w583 w591 w599]
          tunnel: [w572 w580 w588 w596] -> w549
          tunnel: [w571 w579 w587 w595] -> w548
          tunnel: ["A save" "B save" "C save" "D save"] -> w547
          tunnel: [w569 w577 w585 w593] -> w542
          tunnel: [w568 w576 w584 w592] -> w545
          frame "A", Default {
            n284 = local read "A Data 2"() -> (w568:dbl[])
            n285 = local read "A Data"() -> (w569:dbl[])
            n286 = local read "A Array"() -> (w571:string[][])
            n287 = Index Array(array=w575, index (row)=0, index (col)=0 ("disabled index (col)")) -> (element=w572:string)
          }
          frame "B" {
            n288 = local read "B Data 2"() -> (w576:dbl[])
            n289 = local read "B Data"() -> (w577:dbl[])
            n290 = local read "B Array"() -> (w579:string[][])
            n291 = Index Array(array=w583, index (row)=1, index (col)=0 ("disabled index (col)")) -> (element=w580:string)
          }
          frame "C" {
            n292 = local read "C Data 2"() -> (w584:dbl[])
            n293 = local read "C Data"() -> (w585:dbl[])
            n294 = local read "C Array"() -> (w587:string[][])
            n295 = Index Array(array=w591, index (row)=2, index (col)=0 ("disabled index (col)")) -> (element=w588:string)
          }
          frame "D" {
            n296 = local read "D Data 2"() -> (w592:dbl[])
            n297 = local read "D Data"() -> (w593:dbl[])
            n298 = local read "D Array"() -> (w595:string[][])
            n299 = Index Array(array=w599, index (row)=3, index (col)=0 ("disabled index (col)")) -> (element=w596:string)
          }
        }
        n300 = Format Date/Time String(time format string (%c)="%H") -> (date/time string=w559:string)  [unwired: 2 out]
        n301 = Equal?(x=w558, y=w559) -> (x = y?=w555:bool)
        n302 = Equal?(x=w558, y="Backup Hour") -> (x = y?=w554:bool)
        n303 = Not Equal?(x=w542, y=w547) -> (x != y?=w546:bool)
        n304 = Build Array(w542, w545) -> (w544:dbl[][])
        n305 = Format Date/Time String(time format string (%c)="%Y%m%d_%H%M%S_") -> (date/time string=w553:string)  [unwired: 2 out]
        n306 = Not(x=w555) -> (.not. x?=w556:bool)
        n307 = Transpose 2D Array(2D array=w544) -> (transposed array=w543:dbl[][])
        n308 = And(x=w556, y=w554) -> (x .and. y?=w552:bool)
        "robo?" <- w552
        n309 = Concatenate Strings(w553, w551, w536, w549, w536, w535, "_SS_Data.csv" ("string")) -> (w539:string)
        n310 = call "Filename Generate SS.vi"("name or relative path"=w539, "path"=w540) -> ("appended path"=w538:path)  [unwired: 8 in, 1 out]
        n311 = case shown="True" w552 {
          frame False {
          }
          frame True {
            n312 = call <vilib>:"System Exec.vi"("command line"="\"C:\\Program Files\\GE\\Start Stop\\robocopy_backup.bat\"" ("data backup command line")) -> ("error out"=→"Saving":errorcluster)  [unwired: 7 in, 3 out]
          }
        }
        n313 = case shown="True" w546 {
          tunnel: w538 -> [w600 w607]
          tunnel: [w600 w601] -> w561
          tunnel: w548 -> [_ w614]
          tunnel: w543 -> [_ w612]
          tunnel: w535 -> [_ w609]
          tunnel: w542 -> [_ w608]
          tunnel: string[] ["L1 Array, L2 Array(Amps) in 0.5 sec samples, then Com Traffic preceding failure "] ("1D data") -> [_ w605]
          frame False {
          }
          frame True {
            w604 = TRUE ("transpose? (no:F)")
            w611 = "," ("delimiter (\\t)")
            n314 = call-poly <vilib>:"Write To Spreadsheet File.vi"("1D data"=w605, "file path (dialog if empty)"=w607) -> ("new file path (Not A Path if cancelled)"=w606:path)  [unwired: 6 in]
            n315 = case shown="\"D\"" w609 {
              tunnel: w608 -> [w615 w616 w617 w618]
              frame "A", Default {
                n316 = local write "A save"(w615) -> ()
              }
              frame "B" {
                n317 = local write "B save"(w616) -> ()
              }
              frame "C" {
                n318 = local write "C save"(w617) -> ()
              }
              frame "D" {
                n319 = local write "D save"(w618) -> ()
              }
            }
            n320 = call-poly <vilib>:"Write To Spreadsheet File.vi"("delimiter (\\t)"=w611, "transpose? (no:F)"=w604, "append to file? (new file:F)"=w604, "2D data"=w612, "file path (dialog if empty)"=w606) -> ("new file path (Not A Path if cancelled)"=w610:path)  [unwired: 3 in]
            n321 = call-poly <vilib>:"Write To Spreadsheet File.vi"("delimiter (\\t)"=w611, "append to file? (new file:F)"=TRUE, "2D data"=w614, "file path (dialog if empty)"=w610) -> ("new file path (Not A Path if cancelled)"=w602:path)  [unwired: 4 in]
            n322 = Set Permissions(7:i16 0 ("permissions"), 11:w602) -> (3:w601:path)  [unwired: 3 in, 1 out]
          }
        }
        "Current Filename" <- w561
        n323 = Bundle By Name(cluster=w564, "Last Hour"=w559) -> (w563:T8)
        n324 = call <vilib>:"Add State(s) to Queue__jki_lib_state_machine.vi"("State(s) in (\"\")"=w567) -> ("States Out"=w566:string)  [unwired: 14 in]
      }
      frame "Add Select Data" {
        # "Your code here.\n(You can make a copy of, or modify, this frame)"
        n325 = Unbundle By Name(w635) -> ("Label Com Array"=w634:string[][], "UI Array"=w633:T4[])
        n326 = for {
          tunnel: w634 -> [w656] mode=indexing
          tunnel: w633 -> [w651] mode=indexing
          tunnel: [w650] -> w632
          tunnel: [w650] -> w630
          stop <- w652 stop-if-true
          n327 = Unbundle By Name(w651) -> ("Command:Data"=w650:string)
          n328 = Index Array(array=w656, index=0) -> (element=w653:string)
          n329 = Equal?(x=w653, y="Select Station") -> (x = y?=w652:bool)
        }
        n330 = global read "Globals SS.vi" "Max Length of Display Data"() -> (w627:i32)
        n331 = String Length(string=w630) -> (length=w629:i32)
        n332 = Greater Than 0?(x=w629) -> (x > 0?=w628:bool)
        n333 = case shown="True" w628 {
          tunnel: w632 -> [_ w648]
          tunnel: "Command:Data" -> [w639 w647]
          tunnel: [w639 w649] -> w626
          tunnel: w627 -> [_ w641]
          tunnel: "\n--------------------\n" ("string") -> [_ w643]
          frame False {
          }
          frame True {
            n334 = Concatenate Strings(w647, w643, w648) -> (w646:string)
            n335 = String Length(string=w646) -> (length=w645:i32)
            n336 = Subtract(x=w645, y=w641) -> (x-y=w644:i32)
            n337 = In Range and Coerce(upper limit=w641, x=w644, lower limit=0) -> (coerced(x)=w642:i32)  [unwired: 1 out]
            n338 = String Subset(string=w646, offset (0)=w642, length (rest)=w641) -> (substring=w649:string)
          }
        }
        n339 = Search and Replace String(input string=w626, search string="\n") -> (number of replacements=w624:i32)  [unwired: 6 in, 3 out]
        n340 = local write "Command:Data"(w626) -> ()
        n341 = Subtract(x=w624, y=10) -> (x-y=w622:i32)
        n342 = property on="Command:Data" class="Str"("Text.Scroll Position"=w622) -> ()  [unwired: 2 in, 2 out]
        n343 = call <vilib>:"Add State(s) to Queue__jki_lib_state_machine.vi"("State(s) in (\"\")"=w638) -> ("States Out"=w637:string)  [unwired: 14 in]
      }
    }
  }
  "Stop" <- w3
  n344 = while "Gather SS Data State Machine" {
    shift-right: [w660] -> _
    shift-left: _ -> [w659]
    shift-right: [w663] -> _
    shift-left: _ -> [w657]
    shift-right: [w662] -> _
    shift-left: w1 -> [w664]
    stop <- w661 stop-if-true
    w658 = 500  # Timeout
    n345 = call <vilib>:"Parse State Queue__jki_lib_state_machine.vi"("State Queue"=w664, "Error In (no error)"=w657) -> ("Remaining States"=w666:string, "Current State"=w667:string, "Arguments"=w665:string)  [unwired: 11 in]
    n346 = case shown="\"\", \"Idle\"" w667 {
      selector: w667 -> [_ _ w690 _ _ _ _ _ _ _ _ _ _ _ _ _]
      tunnel: w666 -> [w674 w689 w694 w706 w711 w715 w736 w754 w760 w764 w788 w823 w844 w877 w910 w943]
      tunnel: w665 -> [_ _ _ _ _ _ _ _ _ _ _ _ _ _ _ _]
      tunnel: w659 -> [w672 w686 w692 w703 w709 w712 _ w740 w758 w761 w785 w820 w841 w874 w907 w940]
      tunnel: [w671 w687 w696 errorcluster {"status"=FALSE, "code"=0, "source"=""} ("error out") w708 w713 w728 w746 w755 w762 w780 w821 w842 w875 w908 w941] -> w663
      tunnel: w657 -> [w670 w687 w695 w702 w708 w713 w728 w747 w757 w762 w781 w821 w842 w875 w908 w941]
      tunnel: [w673 w688 w693 w705 w710 w714 w735 w753 w759 w763 w787 w822 w843 w876 w909 w942] -> w662
      tunnel: [_ _ _ _ TRUE _ _ _ _ _ _ _ _ _ _ _] -> w661
      tunnel: [w669 w686 w692 w703 w709 w712 w734 w739 w758 w761 w784 w819 w840 w873 w906 w939] -> w660
      tunnel: w658 -> [w668 _ _ _ _ _ _ _ _ _ _ _ _ _ _ _]
      frame "", "Idle" {
        # "executes when the state queue is empty"
        n347 = event shown="[0] Timeout" {
          selector: _ -> [_]
          dyn-events: _ -> [_]
          timeout: w668 -> [_]
          tunnel: w674 -> [w680]
          tunnel: [w679] -> w673
          tunnel: w672 -> [w677]
          tunnel: [w678] -> w671
          tunnel: w670 -> [w678]
          tunnel: [w677] -> w669
          event Timeout {
            n348 = event-data() -> ()  [unwired: 1 in, 1 out]
            n349 = case shown="False" "Change Lint" {
              tunnel: [w682 "" ("State(s) in Front (\"\")")] -> w676
              frame False {
                n350 = local read "Stop"() -> (w681:bool)
                n351 = case shown="False" w681 {
                  tunnel: ["Read Currents\nCheck for Rising Edge\nAdd Data:A\nAdd Data:B\nAdd Data:C\nAdd Data:D\n" ("State(s) in Front (\"\")") "Data: Cleanup\nExit" ("State(s) in Front (\"\")")] -> w682
                  frame False {
                  }
                  frame True {
                  }
                }
              }
              frame True {
              }
            }
            n352 = call <vilib>:"Add State(s) to Queue__jki_lib_state_machine.vi"("State(s) in Front (\"\")"=w676, "State(s) in (\"\")"=w680) -> ("States Out"=w679:string)  [unwired: 13 in]
          }
        }
      }
      frame "---------- Core ----------" {
        # "Do not put any code in this frame.\n(it is a separator no-op)"
        n353 = call <vilib>:"Add State(s) to Queue__jki_lib_state_machine.vi"("State(s) in (\"\")"=w689) -> ("States Out"=w688:string)  [unwired: 14 in]
      }
      frame Default {
        w699 = 42 items=["No error", "Argument error", "Memory is full", "Out of zone", "End of file", "File already open", "Generic file I/O error", "File not found", "File permission error", "Disk is full", "Duplicate path", "Too many files open", "System feature not enabled", "Resource file not found", "Cannot add resource", "Resource not found", "Image not found", "Image memory error", "Pen does not exist", "Config type invalid", "Config token not found", "Config parse error", "Config memory error", "Bad external code format", "Bad external code offset", "External code not present", "Null window", "Destroy window error", "Null menu", "Print aborted", "Bad print record", "Print driver error", "Windows error during printing", "Memory error during printing", "Print dialog error", "Generic print error", "Invalid device refnum", "Device not found", "Device parameter error", "Device unit error", "Cannot open device", "Device call aborted", "Generic error", "Cancelled by user", "Object ID too low", "Object ID too high", "Object not in heap", "Unknown heap", "Unknown object (invalid DefProc)", "Unknown object (DefProc not in table)", "Message out of range", "Invalid (null) method", "Unknown message", "Manager call not supported", "Bad address", "Network operation in progress", "Network operation timed out", "Connection is busy", "Network attribute not supported", "Network error", "Address in use", "System out of memory", "Connection aborted", "Connection refused", "Not connected", "Already connected", "Connection closed", "Initialization error (interapplication manager)", "Bad occurrence", "Wait on unbound occurrence handler", "Occurrence queue overflow", "Datalog type conflict", "Unused", "Unrecognized type (interapplication manager)", "Memory corrupt", "Failed to make temporary DLL", "Old CIN version", "Drag socket not found", "Failed to load drop-object", "Failed to register OLE object", "Failed to release OLE object", "Format specifier type mismatch", "Unknown format specifier", "Too few format specifiers", "Too many format specifiers", "Scan failed", "Newer CIN version", "Error converting to variant", "Runtime menu error", "Password tampered", "Variant attribute not found", "Incompatible variant data type", "Event data is not available", "Event Store is not present", "Occurrence is not found", "Event Queue is not created", "Event info is not available", "Refnum passed is NULL", "Error retrieving Class GUID", "Error retrieving CoClass GUID", "Error retrieving TypeLib GUID.", "Bad built application magic bytes.", "Specific driver is different from the specific driver associated with the Logical Name.", "There is no session opened to the class driver.", "Max Error", "MAX - Error with config objects", "MAX - Error loading configuration", "MAX - Group not supported"]
        # "Current State"
        # "Do not delete, rename, or modify this frame.\n(this is used to capture unhandled states and typos)"
        # "Handle mistyped state name (developer tool)"
        n354 = Format Into String(format string="Software Exception: Unhandled State \"%s\"." ("message"), error in=w695, w690) -> (resulting string=w698:string, error out=w697:errorcluster)  [unwired: 1 in]
        n355 = call <vilib>:"Error Cluster From Error Code.vi"("show call chain? (False)"=TRUE, "error in (no error)"=w697, "error message (\"\")"=w698, "error code (0)"=w699) -> ("error out"=w696:errorcluster)  [unwired: 5 in]
        n356 = call <vilib>:"Add State(s) to Queue__jki_lib_state_machine.vi"("State(s) in (\"\")"=w694) -> ("States Out"=w693:string)  [unwired: 14 in]
      }
      frame "Error Handler" {
        # "Unhandled Error -- Display it"
        # "Handle any errors here.\nYou can also output any states to clean-up after errors occur"
        # "Clear error"
        n357 = call <vilib>:"General Error Handler.vi"("error in (no error)"=w702) -> ()  [unwired: 10 in, 5 out]
        n358 = call <vilib>:"Add State(s) to Queue__jki_lib_state_machine.vi"("State(s) in Front (\"\")"="/* Post Error States", "State(s) in (\"\")"=w706) -> ("States Out"=w705:string)  [unwired: 13 in]
      }
      frame "Exit" {
        # "Do not put any code in this frame.\n(No errors that occur here will be handled.)"
        n359 = call <vilib>:"Add State(s) to Queue__jki_lib_state_machine.vi"("State(s) in (\"\")"=w711) -> ("States Out"=w710:string)  [unwired: 14 in]
      }
      frame "---------- Data ----------" {
        # "Do not put any code in this frame.\n(It is a separator no-op. You can make a copy of this frame to create a new Data frame)"
        n360 = call <vilib>:"Add State(s) to Queue__jki_lib_state_machine.vi"("State(s) in (\"\")"=w715) -> ("States Out"=w714:string)  [unwired: 14 in]
      }
      frame "Data: Initialize" {
        w717 = bool[] [FALSE, FALSE, FALSE, FALSE]  # Rise
        w718 = dbl[] []  # Old Data
        w719 = dbl[] []  # Read Data
        w720 = dbl[] []  # D Data2
        w721 = dbl[] []  # D Data
        w722 = dbl[] []  # C Data2
        w723 = dbl[] []  # C Data
        w724 = dbl[] []  # B Data2
        w725 = dbl[] []  # B Data
        w726 = dbl[] []  # A Data2
        w727 = dbl[] []  # A Data
        w730 = FALSE  # Dlatch
        w731 = FALSE  # Clatch
        w732 = FALSE  # Blatch
        w733 = FALSE  # Alatch
        # "Initialize the shift-register data, here.\n(data names are defined by what you wire into the bundle function)"
        n361 = property on="Waveform Chart" class="WFChart (strict)"("History Data"=dbl[] []) -> ()  [unwired: 2 in, 2 out]
        n362 = Bundle("Alatch"=w733, "Blatch"=w732, "Clatch"=w731, "Dlatch"=w730, "AI Task"="AI Task", "A Data"=w727, "A Data2"=w726, "B Data"=w725, "B Data2"=w724, "C Data"=w723, "C Data2"=w722, "D Data"=w721, "D Data2"=w720, "Read Data"=w719, "Old Data"=w718, "Rise"=w717) -> (w734:T12)  [unwired: 1 in]
        n363 = call <vilib>:"Add State(s) to Queue__jki_lib_state_machine.vi"("State(s) in (\"\")"=w736) -> ("States Out"=w735:string)  [unwired: 14 in]
      }
      frame "Init: AI" {
        w738 = 10083 items=["default"=-1, "RSE"=10083, "NRSE"=10078, "Differential"=10106, "Pseudodifferential"=12529] ("input terminal configuration")
        w750 = 10123 items=["Finite Samples"=10178, "Continuous Samples"=10123] ("sample mode")
        # "3."
        # "2."
        # "1."
        # "Initialize the shift-register data, here.\n(data names are defined by what you wire into the bundle function)"
        n364 = call-poly <vilib>:"DAQmx Create Virtual Channel.vi"("maximum value"="Maximum Value", "minimum value"="Minimum Value", "input terminal configuration"=w738, "physical channels"="AI Channel", "error in"=w747) -> ("task out"=w749:refnum<k21>, "error out"=w748:errorcluster)  [unwired: 9 in]
        n365 = call-poly <vilib>:"DAQmx Timing.vi"("task/channels in"=w749, "sample mode"=w750, "samples per channel"="Samples per Channel", "rate"="Rate", "error in"=w748) -> ("task out"=w751:refnum<k21>, "error out"=w752:errorcluster)  [unwired: 9 in]
        n366 = call <vilib>:"DAQmx Start Task.vi"("task/channels in"=w751, "error in"=w752) -> ("task out"=w741:refnum<k21>, "error out"=w746:errorcluster)  [unwired: 12 in]
        n367 = Bundle By Name(cluster=w740, "AI Task"=w741) -> (w739:T12)
        n368 = call <vilib>:"Add State(s) to Queue__jki_lib_state_machine.vi"("State(s) in (\"\")"=w754) -> ("States Out"=w753:string)  [unwired: 14 in]
      }
      frame "Data: Cleanup" {
        # "Cleanup any data and references, here.\n(this is called automatically, by the Macro: Exit)"
        n369 = Unbundle By Name(w758) -> ("AI Task"=w756:refnum<k21>)
        n370 = call <vilib>:"DAQmx Clear Task.vi"("task in"=w756, "error in"=w757) -> ("error out"=w755:errorcluster)  [unwired: 13 in]
        n371 = call <vilib>:"Add State(s) to Queue__jki_lib_state_machine.vi"("State(s) in (\"\")"=w760) -> ("States Out"=w759:string)  [unwired: 14 in]
      }
      frame "---------- New Category ----------" {
        # "Template Separator\n(You can make a copy of, or modify, this frame)"
        n372 = call <vilib>:"Add State(s) to Queue__jki_lib_state_machine.vi"("State(s) in (\"\")"=w764) -> ("States Out"=w763:string)  [unwired: 14 in]
      }
      frame "Read Currents" {
        w765 = 5.0  # 10V=50A
        # "Your code here.\n(You can make a copy of, or modify, this frame)"
        n373 = Unbundle By Name(w785) -> ("AI Task"=w786:refnum<k21>)
        n374 = call-poly <vilib>:"DAQmx Read.vi"("task/channels in"=w786, "number of samples per channel"=-1, "error in"=w781) -> ("data"=w777:dbl[][], "error out"=w780:errorcluster)  [unwired: 10 in, 1 out]
        "data" <- w777
        n375 = Array Size(array=w777) -> (size(s)=w770:i32[])
        n376 = Multiply Array Elements(1:w770) -> (0:w769:i32)
        n377 = Equal To 0?(x=w769) -> (x = 0?=w768:bool)
        n378 = case shown="True" w768 {
          tunnel: [_ "Read Currents" ("State(s) in Front (\"\")")] -> w767
          frame False {
          }
          frame True {
          }
        }
        n379 = Index Array(array=w770, index=1) -> (element=w775:i32)
        n380 = Decrement(x=w775) -> (x-1=w771:i32)
        n381 = Delete From Array(array=w777, length=1, index (col)=w771) -> (deleted portion=w773:dbl[][])  [unwired: 1 in, 1 out]
        n382 = Reshape Array(w773, 8 ("dimension size")) -> (w772:dbl[])
        n383 = Multiply(x=w765, y=w772) -> (x*y=w766:dbl[])
        "Currents" <- w766
        n384 = Bundle By Name(cluster=w785, "Read Data"=w766) -> (w784:T12)
        n385 = Index Array(array=w766, index="Channel") -> (element=→"Waveform Chart":dbl)
        n386 = call <vilib>:"Add State(s) to Queue__jki_lib_state_machine.vi"("State(s) in Front (\"\")"=w767, "State(s) in (\"\")"=w788) -> ("States Out"=w787:string)  [unwired: 13 in]
      }
      frame "Check for Rising Edge" {
        n387 = Unbundle By Name(w820) -> ("Read Data"=w818:dbl[], "Old Data"=w817:dbl[], "A Data"=w809:dbl[], "B Data"=w808:dbl[], "C Data"=w807:dbl[], "D Data"=w806:dbl[])
        n388 = Array Size(array=w807) -> (size(s)=w803:i32)
        n389 = Array Size(array=w809) -> (size(s)=w805:i32)
        n390 = local read "Max Len"() -> (w790:i32)
        n391 = Array Size(array=w806) -> (size(s)=w802:i32)
        n392 = Array Size(array=w808) -> (size(s)=w804:i32)
        n393 = Build Array(w805, w804, w803, w802) -> (w801:i32[])
        n394 = In Range and Coerce(upper limit=w790, x=w801, lower limit=0 ("Max Len of Cyc")) -> (In Range?=w800:bool[])  [unwired: 1 out]
        n395 = Not(x=w800) -> (.not. x?=w799:bool[])
        n396 = global read "Globals SS.vi" "A L1 Index"() -> (w813:i32)
        n397 = global read "Globals SS.vi" "B L1 index"() -> (w812:i32)
        n398 = global read "Globals SS.vi" "D L1 index"() -> (w810:i32)
        n399 = global read "Globals SS.vi" "C L1 index"() -> (w811:i32)
        n400 = Less Or Equal?(x=w817, y="Off On Threshold") -> (x <= y?=w816:bool[])
        n401 = Greater?(x=w818, y="Off On Threshold") -> (0:w815:bool[])
        n402 = And(x=w816, y=w815) -> (x .and. y?=w814:bool[])
        n403 = Index Array(array=w814, index #1=w813, index #2=w812, index #3=w811, index #4=w810) -> (element #1=w798:bool, element #2=w797:bool, element #3=w796:bool, element #4=w795:bool)
        n404 = Build Array(w798, w797, w796, w795) -> (w794:bool[])
        n405 = Compound Arithmetic op=AND(w794, w799) -> (w793:bool[])
        n406 = Bundle By Name(cluster=w820, "Old Data"=w818, "Rise"=w793) -> (w819:T12)
        n407 = call "Rising Edge Latch.vi"("S Rising Edge"=w793) -> ()  [unwired: 10 in, 1 out]
        n408 = call <vilib>:"Add State(s) to Queue__jki_lib_state_machine.vi"("State(s) in (\"\")"=w823) -> ("States Out"=w822:string)  [unwired: 14 in]
      }
      frame "Add Data:A" {
        n409 = Unbundle By Name(w841) -> ("Read Data"=w837:dbl[], "A Data"=w835:dbl[], "A Data2"=w834:dbl[], "Alatch"=w833:bool, "Rise"=w827:bool[])
        n410 = Array To Cluster(array=w827) -> (cluster=w832:T13)
        n411 = global read "Globals SS.vi" "A L1 Index"() -> (w839:i32)
        n412 = global read "Globals SS.vi" "A L2 Index"() -> (w838:i32)
        n413 = Unbundle(w832) -> ("Rise[0]"=w831:bool)  [unwired: 3 out]
        n414 = Index Array(array=w837, index #1=w839, index #2=w838) -> (element #1=w830:dbl, element #2=w829:dbl)
        n415 = local read "Max Len"() -> (w824:i32)
        n416 = Or(x=w831, y=w833) -> (x .or. y?=w828:bool)
        n417 = case shown="True" w828 {
          tunnel: w831 -> [_ w851]
          tunnel: w835 -> [w847 w856]
          tunnel: [w847 w855] -> w826
          tunnel: w830 -> [_ w854]
          tunnel: [w846 w853] -> w825
          tunnel: w834 -> [w846 w852]
          tunnel: w829 -> [_ w850]
          tunnel: w824 -> [_ w849]
          tunnel: [w845 TRUE ("Alatch")] -> w836
          tunnel: w833 -> [w845 _]
          frame False {
          }
          frame True {
            n418 = call "Add val to Array w Limit.vi"("size limit"=w849, "Value"=w850, "Array In"=w852, "Init?"=w851) -> ("Array  Out"=w853:dbl[])  [unwired: 7 in]
            n419 = call "Add val to Array w Limit.vi"("size limit"=w849, "Value"=w854, "Array In"=w856, "Init?"=w851) -> ("Array  Out"=w855:dbl[])  [unwired: 7 in]
          }
        }
        n420 = Bundle By Name(cluster=w841, "Alatch"=w836, "A Data"=w826, "A Data2"=w825) -> (w840:T12)
        n421 = local write "A Data 2"(w825) -> ()
        n422 = local write "A Data"(w826) -> ()
        n423 = call <vilib>:"Add State(s) to Queue__jki_lib_state_machine.vi"("State(s) in (\"\")"=w844) -> ("States Out"=w843:string)  [unwired: 14 in]
      }
      frame "Add Data:B" {
        n424 = Unbundle By Name(w874) -> ("Read Data"=w870:dbl[], "B Data"=w868:dbl[], "B Data2"=w867:dbl[], "Blatch"=w866:bool, "Rise"=w861:bool[])
        n425 = Array To Cluster(array=w861) -> (cluster=w865:T13)
        n426 = global read "Globals SS.vi" "B L1 index"() -> (w872:i32)
        n427 = global read "Globals SS.vi" "B L2 index"() -> (w871:i32)
        n428 = Unbundle(w865) -> ("Rise[1]"=w860:bool)  [unwired: 3 out]
        n429 = Index Array(array=w870, index #1=w872, index #2=w871) -> (element #1=w864:dbl, element #2=w863:dbl)
        n430 = local read "Max Len"() -> (w857:i32)
        n431 = Or(x=w860, y=w866) -> (x .or. y?=w862:bool)
        n432 = case shown="True" w862 {
          tunnel: w860 -> [_ w884]
          tunnel: w868 -> [w880 w889]
          tunnel: [w880 w888] -> w859
          tunnel: w864 -> [_ w887]
          tunnel: [w879 w886] -> w858
          tunnel: w867 -> [w879 w885]
          tunnel: w863 -> [_ w883]
          tunnel: w857 -> [_ w882]
          tunnel: [w878 TRUE ("Alatch")] -> w869
          tunnel: w866 -> [w878 _]
          frame False {
          }
          frame True {
            n433 = call "Add val to Array w Limit.vi"("size limit"=w882, "Value"=w883, "Array In"=w885, "Init?"=w884) -> ("Array  Out"=w886:dbl[])  [unwired: 7 in]
            n434 = call "Add val to Array w Limit.vi"("size limit"=w882, "Value"=w887, "Array In"=w889, "Init?"=w884) -> ("Array  Out"=w888:dbl[])  [unwired: 7 in]
          }
        }
        n435 = Bundle By Name(cluster=w874, "Blatch"=w869, "B Data"=w859, "B Data2"=w858) -> (w873:T12)
        n436 = local write "B Data 2"(w858) -> ()
        n437 = local write "B Data"(w859) -> ()
        n438 = call <vilib>:"Add State(s) to Queue__jki_lib_state_machine.vi"("State(s) in (\"\")"=w877) -> ("States Out"=w876:string)  [unwired: 14 in]
      }
      frame "Add Data:C" {
        n439 = Unbundle By Name(w907) -> ("Read Data"=w903:dbl[], "C Data"=w901:dbl[], "C Data2"=w900:dbl[], "Clatch"=w899:bool, "Rise"=w894:bool[])
        n440 = Array To Cluster(array=w894) -> (cluster=w898:T13)
        n441 = global read "Globals SS.vi" "C L1 index"() -> (w905:i32)
        n442 = global read "Globals SS.vi" "C L2 index"() -> (w904:i32)
        n443 = Unbundle(w898) -> ("Rise[2]"=w893:bool)  [unwired: 3 out]
        n444 = Index Array(array=w903, index #1=w905, index #2=w904) -> (element #1=w897:dbl, element #2=w896:dbl)
        n445 = local read "Max Len"() -> (w890:i32)
        n446 = Or(x=w893, y=w899) -> (x .or. y?=w895:bool)
        n447 = case shown="True" w895 {
          tunnel: w893 -> [_ w917]
          tunnel: w901 -> [w913 w922]
          tunnel: [w913 w921] -> w892
          tunnel: w897 -> [_ w920]
          tunnel: [w912 w919] -> w891
          tunnel: w900 -> [w912 w918]
          tunnel: w896 -> [_ w916]
          tunnel: w890 -> [_ w915]
          tunnel: [w911 TRUE ("Alatch")] -> w902
          tunnel: w899 -> [w911 _]
          frame False {
          }
          frame True {
            n448 = call "Add val to Array w Limit.vi"("size limit"=w915, "Value"=w916, "Array In"=w918, "Init?"=w917) -> ("Array  Out"=w919:dbl[])  [unwired: 7 in]
            n449 = call "Add val to Array w Limit.vi"("size limit"=w915, "Value"=w920, "Array In"=w922, "Init?"=w917) -> ("Array  Out"=w921:dbl[])  [unwired: 7 in]
          }
        }
        n450 = local write "C Data 2"(w891) -> ()
        n451 = Bundle By Name(cluster=w907, "Clatch"=w902, "C Data"=w892, "C Data2"=w891) -> (w906:T12)
        n452 = local write "C Data"(w892) -> ()
        n453 = call <vilib>:"Add State(s) to Queue__jki_lib_state_machine.vi"("State(s) in (\"\")"=w910) -> ("States Out"=w909:string)  [unwired: 14 in]
      }
      frame "Add Data:D" {
        n454 = Unbundle By Name(w940) -> ("Read Data"=w936:dbl[], "D Data"=w934:dbl[], "D Data2"=w933:dbl[], "Dlatch"=w932:bool, "Rise"=w927:bool[])
        n455 = Array To Cluster(array=w927) -> (cluster=w931:T13)
        n456 = global read "Globals SS.vi" "D L1 index"() -> (w938:i32)
        n457 = global read "Globals SS.vi" "D L2 index"() -> (w937:i32)
        n458 = Unbundle(w931) -> ("Rise[3]"=w926:bool)  [unwired: 3 out]
        n459 = Index Array(array=w936, index #1=w938, index #2=w937) -> (element #1=w930:dbl, element #2=w929:dbl)
        n460 = Or(x=w926, y=w932) -> (x .or. y?=w928:bool)
        n461 = local read "Max Len"() -> (w923:i32)
        n462 = case shown="True" w928 {
          tunnel: w926 -> [_ w950]
          tunnel: w934 -> [w946 w955]
          tunnel: [w946 w954] -> w925
          tunnel: w930 -> [_ w953]
          tunnel: [w945 w952] -> w924
          tunnel: w933 -> [w945 w951]
          tunnel: w929 -> [_ w949]
          tunnel: w923 -> [_ w948]
          tunnel: [w944 TRUE ("Alatch")] -> w935
          tunnel: w932 -> [w944 _]
          frame False {
          }
          frame True {
            n463 = call "Add val to Array w Limit.vi"("size limit"=w948, "Value"=w953, "Array In"=w955, "Init?"=w950) -> ("Array  Out"=w954:dbl[])  [unwired: 7 in]
            n464 = call "Add val to Array w Limit.vi"("size limit"=w948, "Value"=w949, "Array In"=w951, "Init?"=w950) -> ("Array  Out"=w952:dbl[])  [unwired: 7 in]
          }
        }
        n465 = Bundle By Name(cluster=w940, "Dlatch"=w935, "D Data"=w925, "D Data2"=w924) -> (w939:T12)
        n466 = local write "D Data 2"(w924) -> ()
        n467 = local write "D Data"(w925) -> ()
        n468 = call <vilib>:"Add State(s) to Queue__jki_lib_state_machine.vi"("State(s) in (\"\")"=w943) -> ("States Out"=w942:string)  [unwired: 14 in]
      }
    }
  }
  n469 = property on="Stop" class="Bool (strict)"("Val(Sgnl)"=w3) -> ()  [unwired: 2 in, 2 out]
